vi "HV_Analyse.vi"() -> ()   [LabVIEW 2018]
uses:
  <vilib>/Utility/file.llb/Read Delimited Spreadsheet (string).vi
  <vilib>/Analysis/NI_AALPro.lvlib
panel:
  in  "Main":T1(tab)
  in  "Sow_Median_L1":bool caption="Checkbox"
  out "Progress":dbl(slide) scale=0.0..100.0
  in  "Start":bool
  in  "File path":path
  in  "Threshold [uA]":dbl=0.05
  in  "Window size [min]":dbl=2.0 min=2.0 max=180.0 step=1.0
  in  "Stop":bool
  out "L1-Voltage":cluster{timestamp[], dbl[]}[](graph)
  out "L1-Current [uA]":T2(graph)
  out "L1-Average/WindowSize":T3(graph)
  out "L1-Sparks/min":T4(graph)
  in  "Sow_Median_L2":bool caption="Checkbox"
  out "L2-Sparks/min":T4(graph)
  out "L2-Average/WindowSize":T3(graph)
  out "L2-Current [uA]":T2(graph)
  out "L2-Voltage":cluster{timestamp[], dbl[]}[](graph)
  in  "Sow_Median_L3":bool caption="Checkbox"
  out "L3-Voltage":cluster{timestamp[], dbl[]}[](graph)
  out "L3-Current [uA]":T2(graph)
  out "L3-Average/WindowSize":T3(graph)
  out "L3-Sparks/min":T4(graph)
  in  "Sow_Median_L4":bool caption="Checkbox"
  out "L4-Sparks/min":T4(graph)
  out "L4-Average/WindowSize":T3(graph)
  out "L4-Current [uA]":T2(graph)
  out "L4-Voltage":cluster{timestamp[], dbl[]}[](graph)
  out "Spark-rate statistic_L4":T5(graph) caption="XY Graph - Dark"
  out "Spark-rate statistic_L3":T5(graph) caption="XY Graph - Dark"
  out "Spark-rate statistic_L2":T5(graph) caption="XY Graph - Dark"
  out "Spark-rate statistic_L1":T5(graph) caption="XY Graph - Dark"
  in  "L4_Vertical Slider":cluster{"Slider":dbl, "Slider":dbl}(slide)={"Slider"=0.0, "Slider"=6.702127659574468} scale=-0.25..1.0
  in  "L4_Horizontal Slider":cluster{"Slider":dbl, "Slider":dbl}(slide)={"Slider"=0.0, "Slider"=2.46031746031746} scale=3644665200.0..3644907785.0 scale format="%<%H:%M:%S>T"
  out "L4-Current_Zoomed":cluster{timestamp[], dbl[]}[](graph)
  out "L4-Current_Full":cluster{timestamp[], dbl[]}[](graph)
  in  "L3_Vertical Slider":cluster{"Slider":dbl, "Slider":dbl}(slide)={"Slider"=0.0, "Slider"=6.702127659574468} scale=-1.0..3.0
  in  "L3_Horizontal Slider":cluster{"Slider":dbl, "Slider":dbl}(slide)={"Slider"=0.0, "Slider"=2.46031746031746} scale=3644665200.0..3644907785.0 scale format="%<%H:%M:%S>T"
  out "L3-Current_Zoomed":cluster{timestamp[], dbl[]}[](graph)
  out "L3-Current_Full":cluster{timestamp[], dbl[]}[](graph)
  in  "L2_Vertical Slider":cluster{"Slider":dbl, "Slider":dbl}(slide)={"Slider"=0.0, "Slider"=6.702127659574468} scale=-50.0..100.0
  in  "L2_Horizontal Slider":cluster{"Slider":dbl, "Slider":dbl}(slide)={"Slider"=0.0, "Slider"=2.46031746031746} scale=3644665200.0..3644907785.0 scale format="%<%H:%M:%S>T"
  out "L2-Current_Zoomed":cluster{timestamp[], dbl[]}[](graph)
  out "L2-Current_Full":cluster{timestamp[], dbl[]}[](graph)
  in  "L1_Vertical Slider":cluster{"Slider":dbl, "Slider":dbl}(slide)={"Slider"=0.0, "Slider"=6.702127659574468} scale=-0.2..0.8 scale format="%#_3f"
  in  "L1_Horizontal Slider":cluster{"Slider":dbl, "Slider":dbl}(slide)={"Slider"=0.0, "Slider"=2.46031746031746} scale=3644665200.0..3644907785.0 scale format="%<%H:%M:%S>T"
  out "L1-Current_Zoomed":cluster{timestamp[], dbl[]}[](graph)
  out "L1-Current_Full":cluster{timestamp[], dbl[]}[](graph)
  # "%"
  # "show Median"
  # "show Median"
  # "show Median"
  # "show Median"
  # "Current [uA]"
  # "Current [uA]"
  # "Time"
  # "Time"
  # "Current [uA]"
  # "Current [uA]"
  # "Time"
  # "Time"
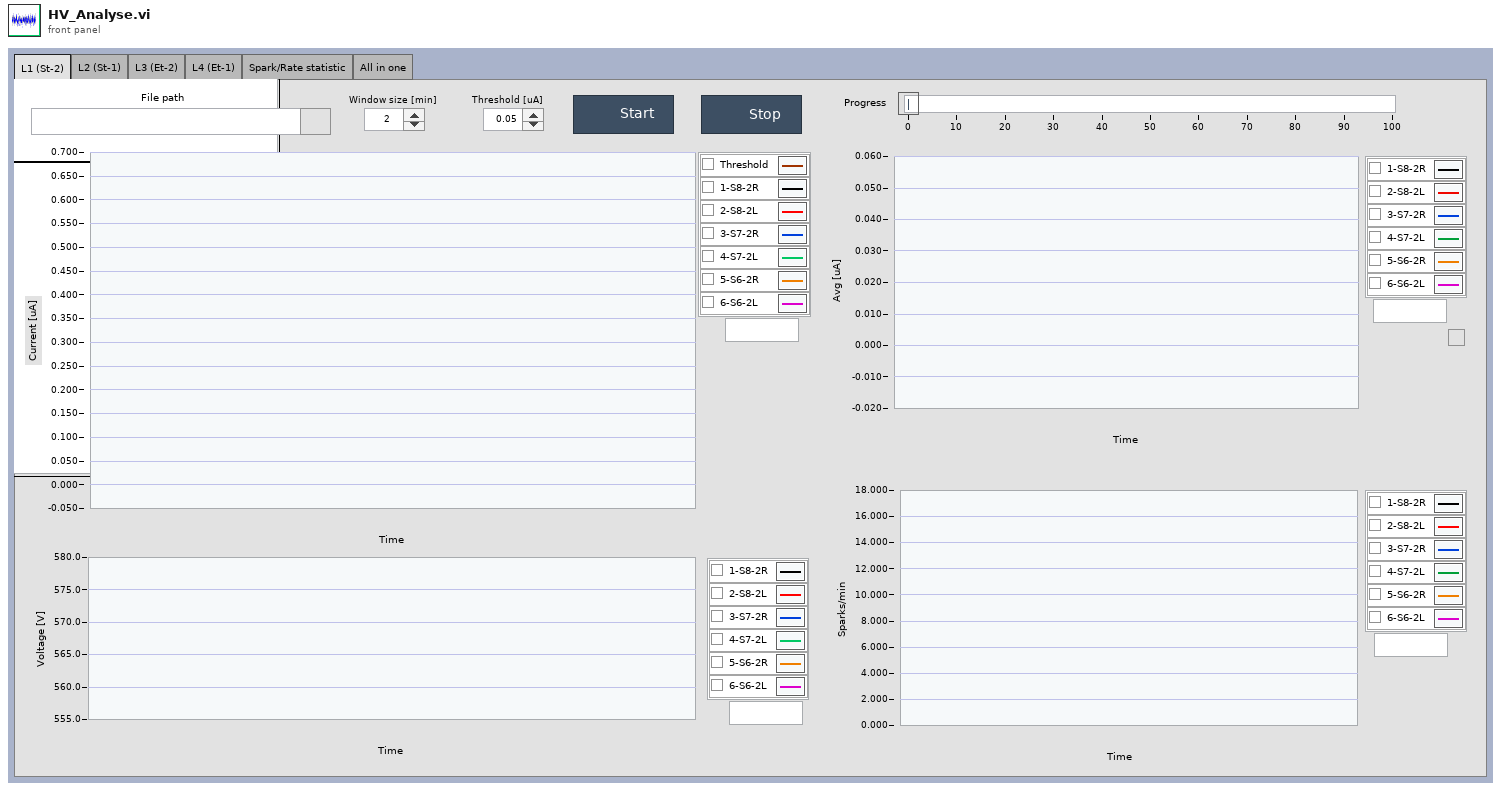
[diagram p1: front panel]
types:
  T1 = enum32{"L1 (St-2)", "L2 (St-1)", "L3 (Et-2)", "L4 (Et-1)", "Spark/Rate statistic", "All in one"}
  T2 = cluster{"Time_Stamp":timestamp[], "Current_Out":dbl[]}[]
  T3 = cluster{"Time_Out":timestamp[], "Window_Avg_OUT":dbl[]}[]
  T4 = cluster{"Time_Out":timestamp[], "Window_Spark_Rate_OUT":dbl[]}[]
  T5 = cluster{"X Values":dbl[], "Histogram: h(x)":i32[]}[]
  T6 = typedef "LVDateTimeRec.ctl" = cluster{"fractional second":dbl, "second":i32, "minute":i32, "hour":i32, "day of month":i32, "month":i32, "year":i32, "day of week":i32, "day of year":i32, "DST":i32}
  T7 = cluster{dbl, i32, i32, i32, "day of month":i32, "month":i32, "year":i32, "day of week":i32, "day of year":i32, "DST":i32}
  T8 = cluster{"XScale.Maximum":dbl, "XScale.Minimum":dbl}
  T9 = cluster{"YScale.Maximum":dbl, "YScale.Minimum":dbl}
  T10 = cluster{"X Values":dbl[], "Histogram: h(x)":i32[]}
  T11 = cluster{"Time_Out":timestamp[], "Window_Avg_OUT":dbl[]}
  T12 = cluster{"Time_Out":timestamp[], "Window_Spark_Rate_OUT":dbl[]}
  T13 = cluster{"Time_Out":timestamp[], "Window_Median_OUT":dbl[]}
  T14 = cluster{"Time_Out":timestamp[], "Window_Median_OUT":dbl[]}[]
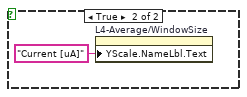
[diagram p3: hidden frame]
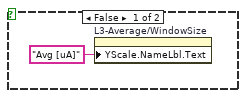
[diagram p4: hidden frame]
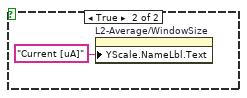
[diagram p5: hidden frame]
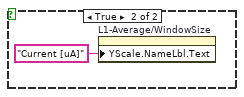
[diagram p6: hidden frame]
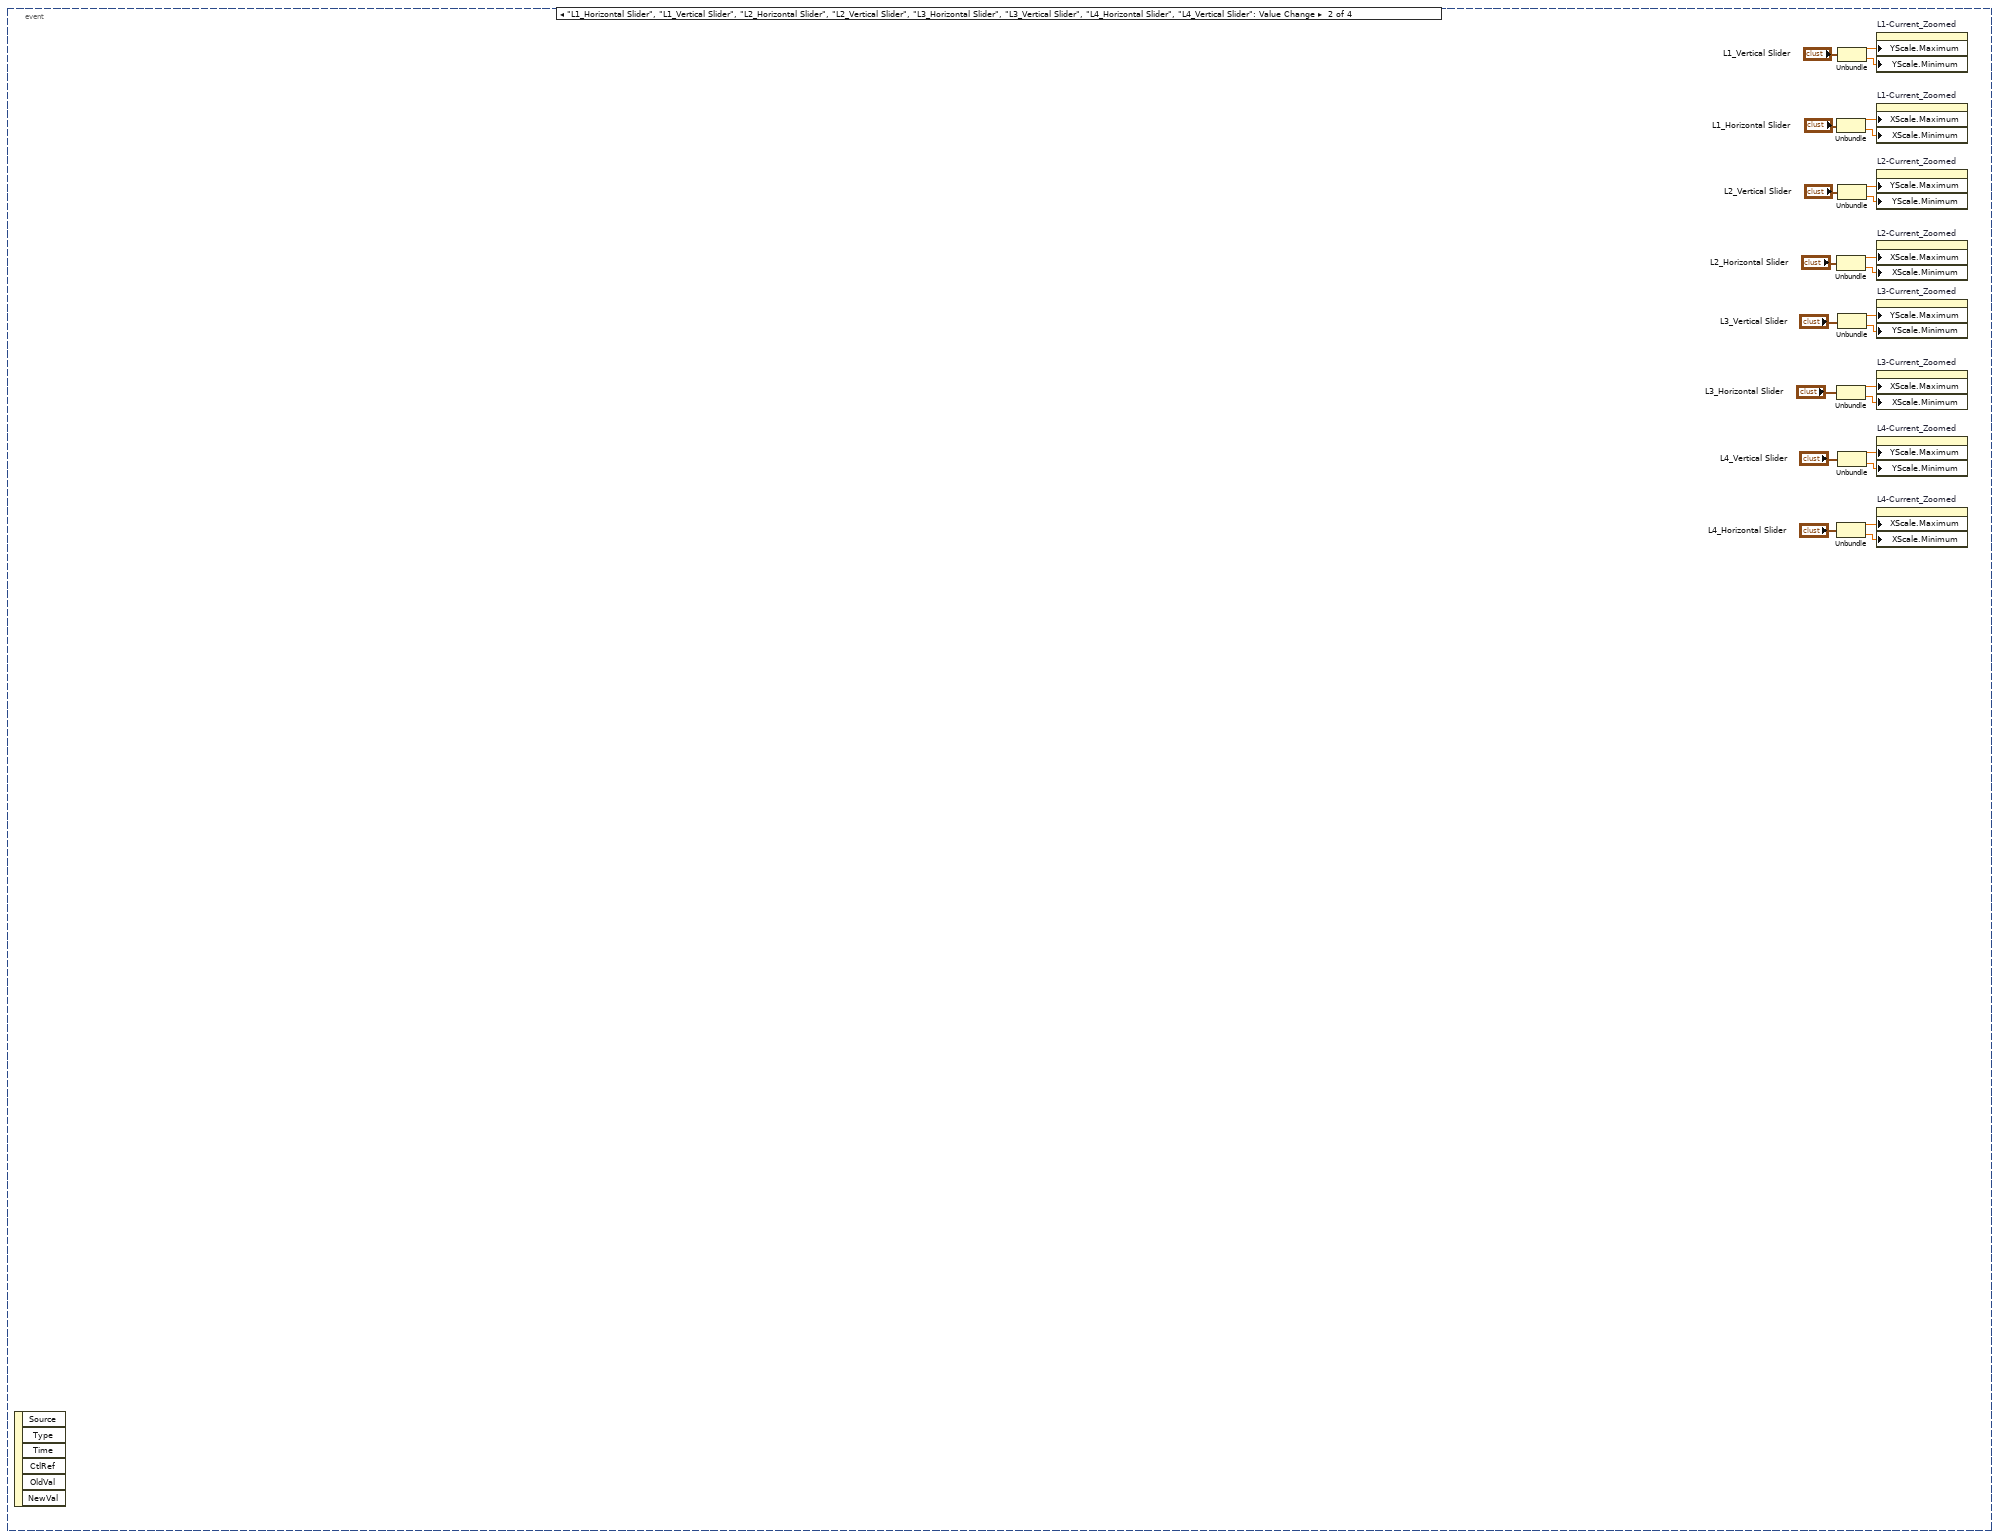
[diagram p7: hidden frame]
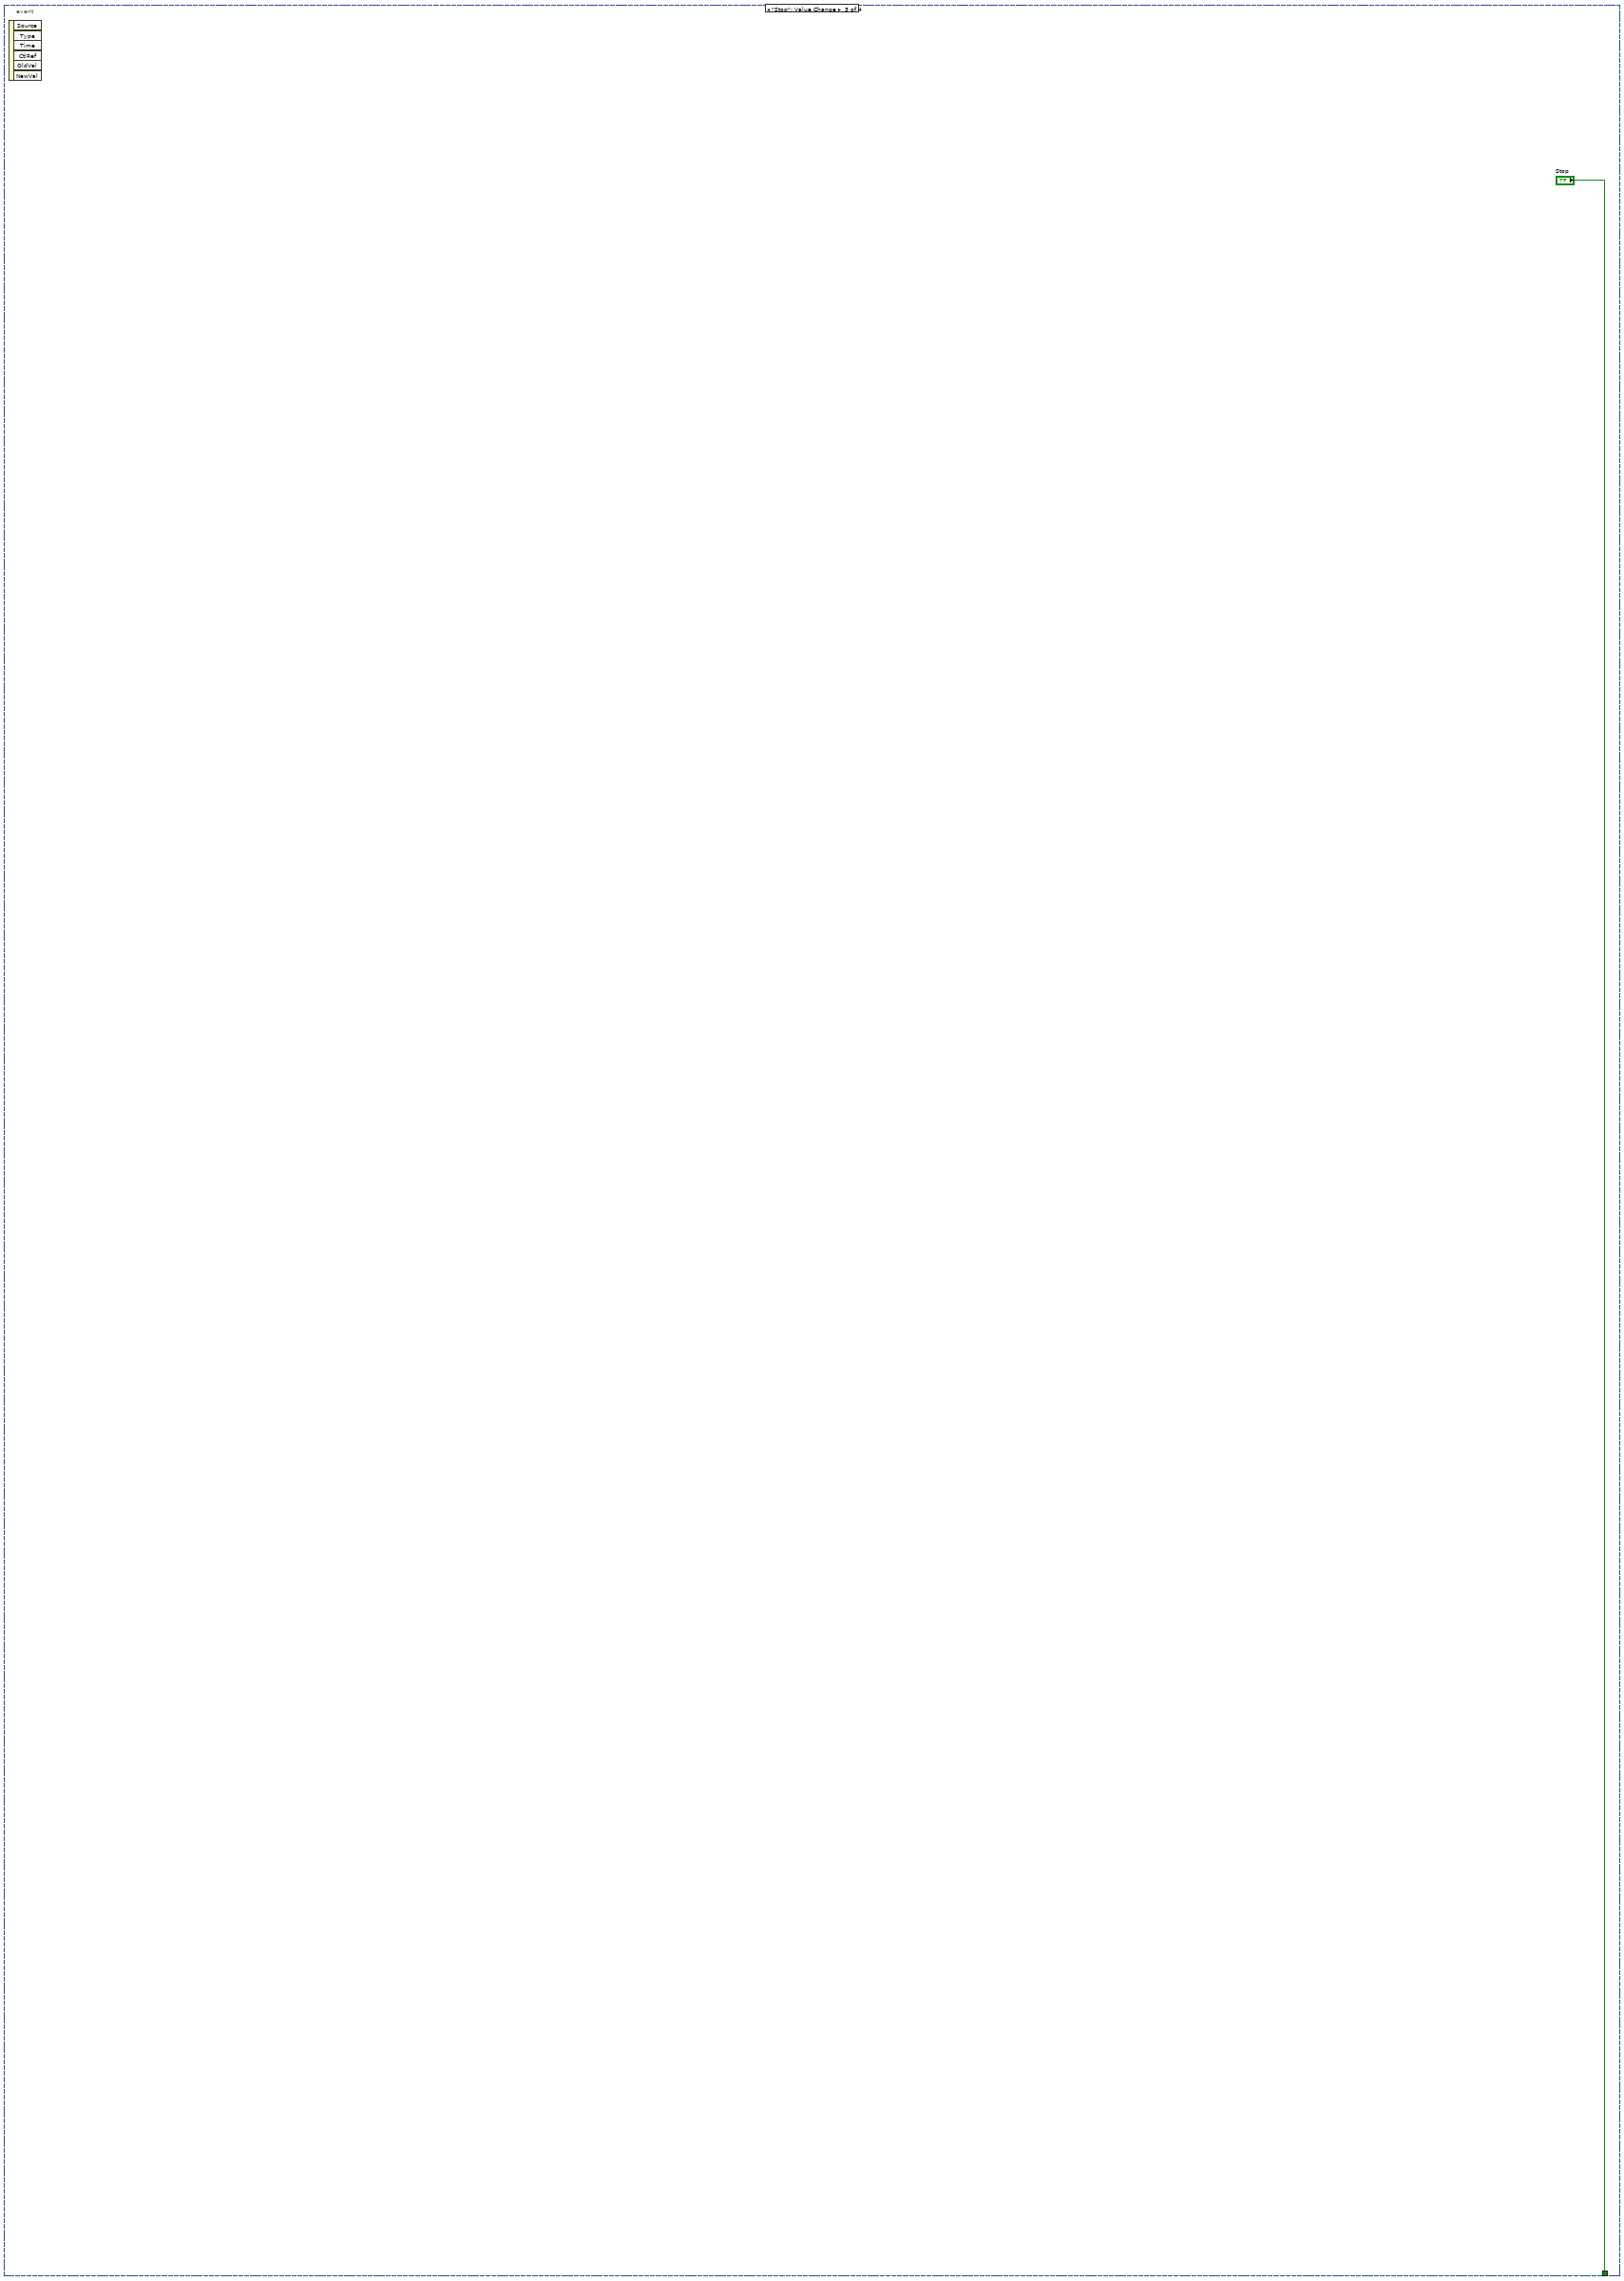
[diagram p8: hidden frame]
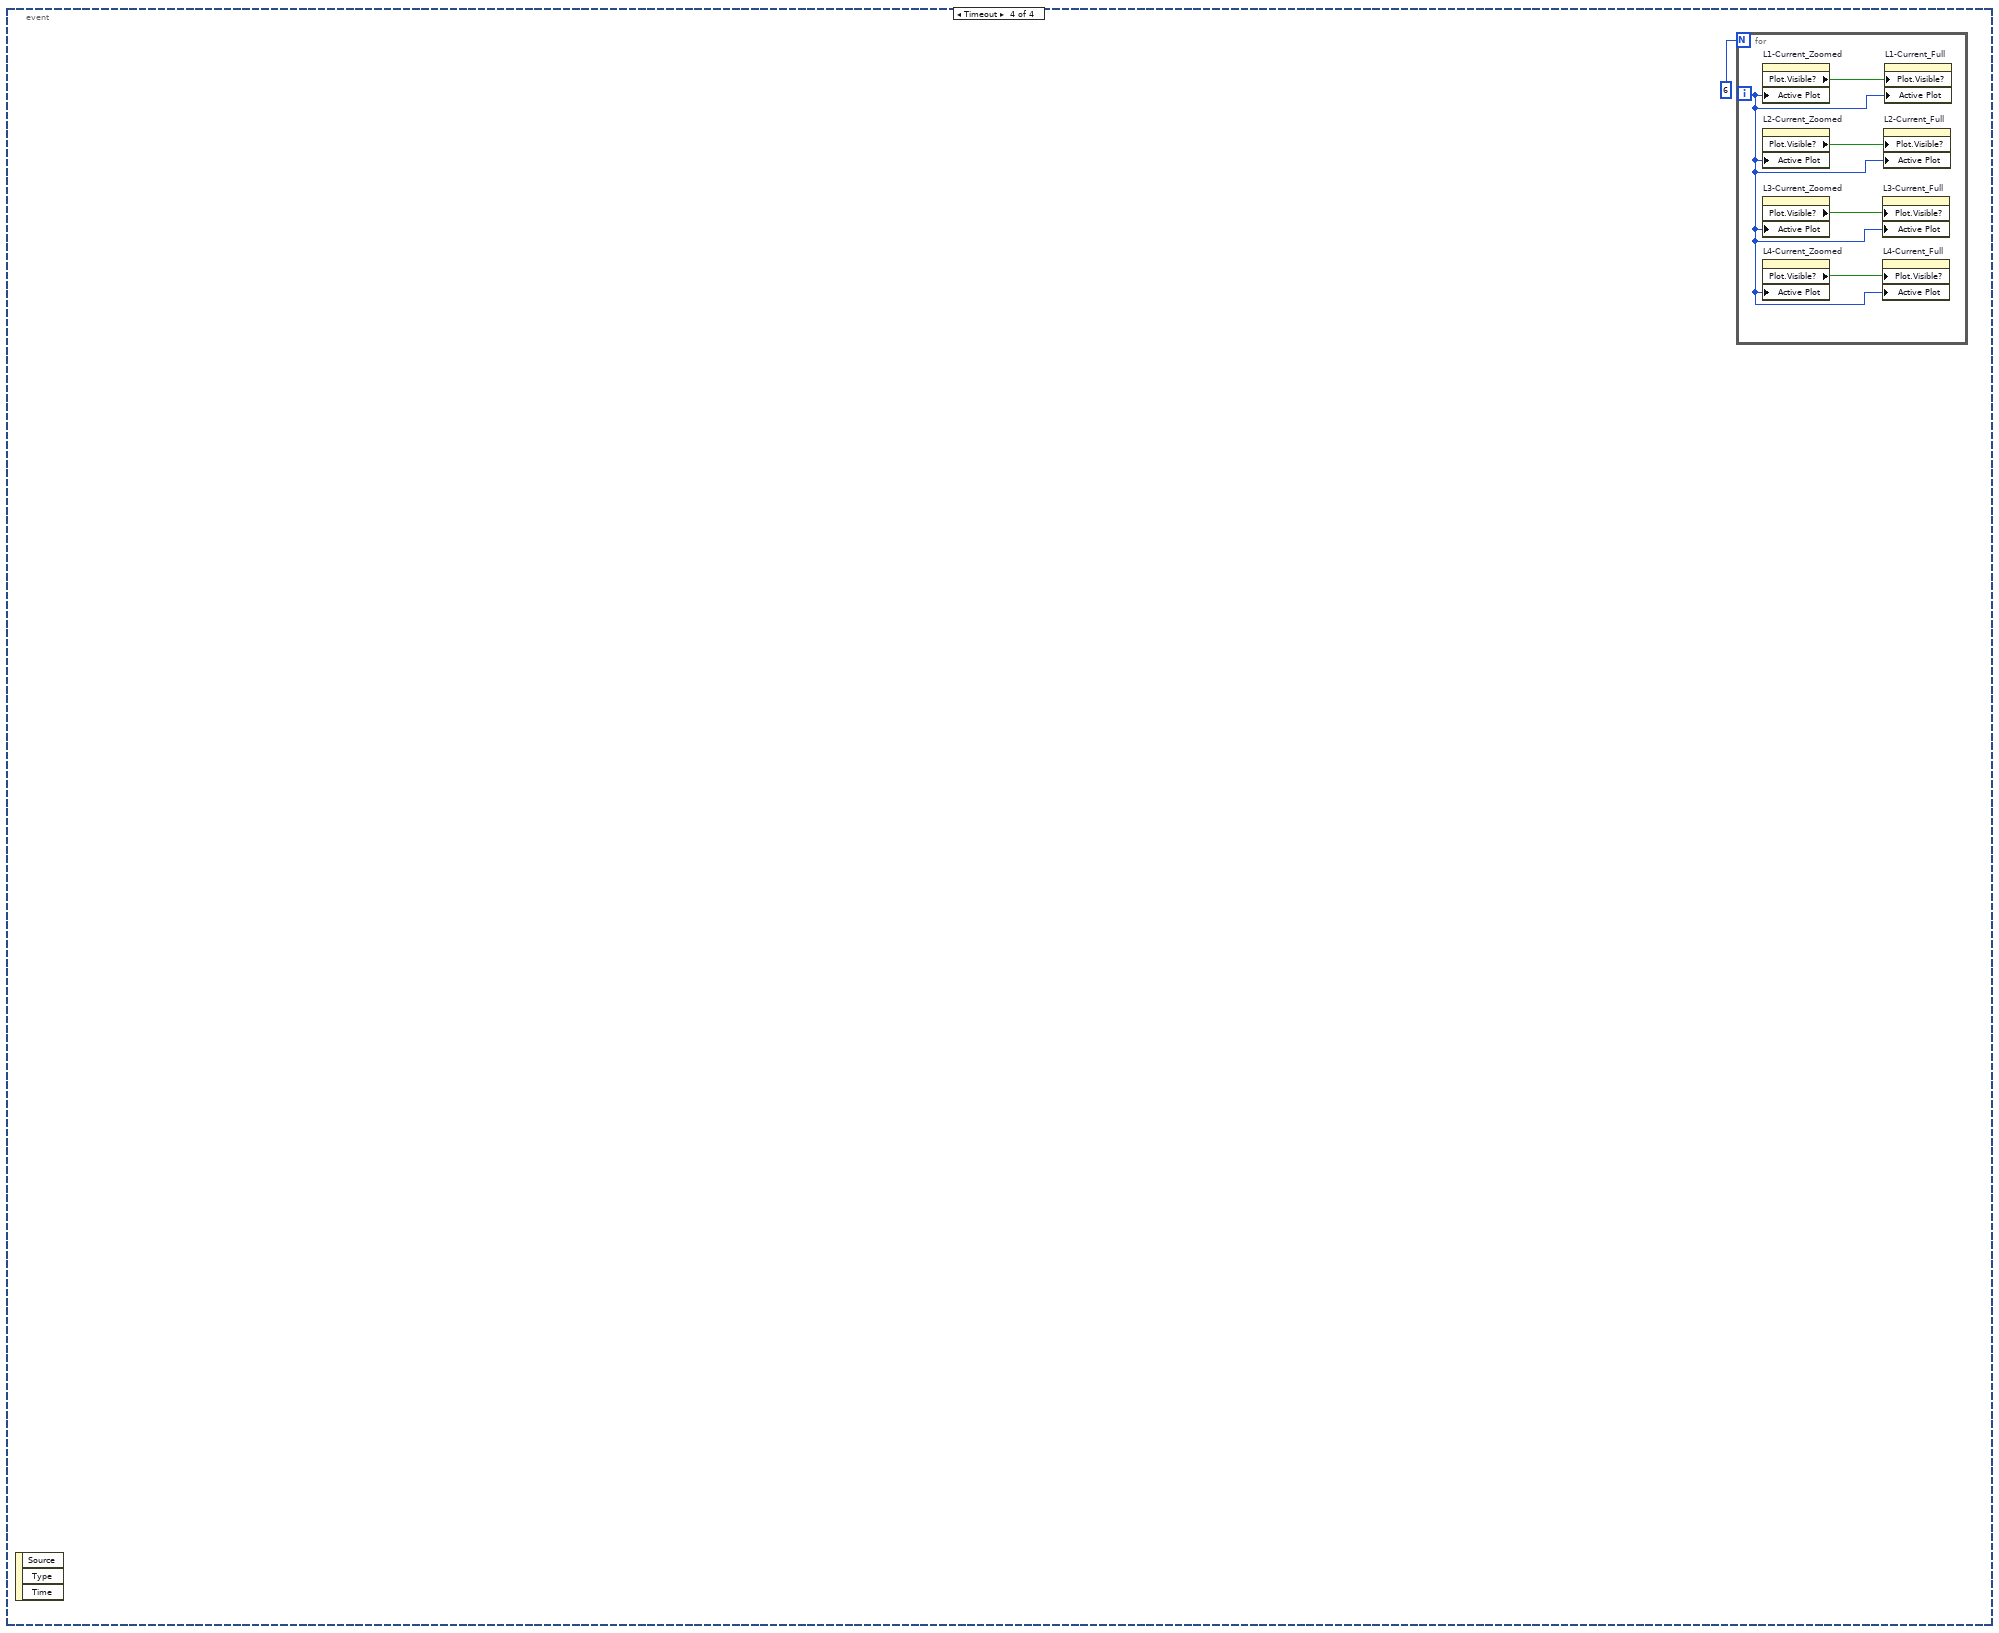
[diagram p9: hidden frame]
diagram:
  n1 = while {
    stop <- w1 stop-if-true
    n2 = event shown="[0] \"Start\", \"Sow_Median_L1\", \"Sow_Median_L2\", \"Sow_Median_L3\", \"Sow_Median_L4\": Value Change" {
      selector: _ -> [_ _ _ _]
      dyn-events: _ -> [_ _ _ _]
      timeout: 400 -> [_ _ _ _]
      tunnel: [_ _ "Stop" _] -> w1
      event "Start", "Sow_Median_L1", "Sow_Median_L2", "Sow_Median_L3", "Sow_Median_L4": Value Change {
        w385 = 31 ("# bins")
        w387 = 0.0 ("min")
        w386 = 6.2 ("max")
        w412 = 31 ("# bins")
        w410 = 0.0 ("min")
        w411 = 6.2 ("max")
        w683 = 0
        # "Amount of windows size"
        # "Full time in minute"
        # "Full time in seconds"
        # "First time stamp"
        # "Last time stamp"
        # "Ch24"
        # "Ch23"
        # "Ch22"
        # "Ch21"
        # "Ch20"
        # "Ch19"
        # "Ch18"
        # "Ch17"
        # "Ch16"
        # "Ch15"
        # "Ch14"
        # "Ch13"
        # "Ch12"
        # "Ch11"
        # "Ch10"
        # "Ch9"
        # "Ch8"
        # "Ch7"
        # "Ch6"
        # "Ch5"
        # "Ch4"
        # "Ch3"
        # "Ch2"
        # "Ch1"
        # "Ch19-Ch24\nCurrent"
        # "Ch13-Ch18\nCurrent"
        # "Ch7-Ch12\nCurrent"
        # "Ch1-Ch6\nCurrent"
        # "Graphs for slider\nmanipulation"
        # "Time Stamp array"
        # "Threshold Graph\nIndicator"
        # "Vlotage Graphs"
        # "L4"
        # "L3"
        # "L2"
        # "L1"
        n3 = event-data() -> ()  [unwired: 1 in, 6 out]
        n4 = call-poly <vilib>:"Read Delimited Spreadsheet.vi"("file path (dialog if empty)"="File path") -> ("all rows"=w112:string[][])  [unwired: 9 in, 5 out]
        n5 = Index Array(array=w112, index (col)=0 ("disabled index (col)")) -> (element=w354:string[])  [unwired: 1 in]
        n6 = Index Array(array=w112, index (col)=1 ("disabled index (col)")) -> (element=w350:string[])  [unwired: 1 in]
        n7 = Index Array(array=w112, index (col)=2 ("disabled index (col)")) -> (element=w345:string[])  [unwired: 1 in]
        n8 = Index Array(array=w112, index (col)=5 ("disabled index (col)")) -> (element=w316:string[])  [unwired: 1 in]
        n9 = Index Array(array=w112, index (col)=6 ("disabled index (col)")) -> (element=w321:string[])  [unwired: 1 in]
        n10 = Index Array(array=w112, index (col)=15 ("disabled index (col)")) -> (element=w275:string[])  [unwired: 1 in]
        n11 = Index Array(array=w112, index (col)=16 ("disabled index (col)")) -> (element=w280:string[])  [unwired: 1 in]
        n12 = Index Array(array=w112, index (col)=25 ("disabled index (col)")) -> (element=w309:string[])  [unwired: 1 in]
        n13 = Index Array(array=w112, index (col)=26 ("disabled index (col)")) -> (element=w304:string[])  [unwired: 1 in]
        n14 = Index Array(array=w112, index (col)=3 ("disabled index (col)")) -> (element=w336:string[])  [unwired: 1 in]
        n15 = Index Array(array=w112, index (col)=4 ("disabled index (col)")) -> (element=w340:string[])  [unwired: 1 in]
        n16 = Index Array(array=w112, index (col)=13 ("disabled index (col)")) -> (element=w331:string[])  [unwired: 1 in]
        n17 = Index Array(array=w112, index (col)=14 ("disabled index (col)")) -> (element=w326:string[])  [unwired: 1 in]
        n18 = Index Array(array=w112, index (col)=17 ("disabled index (col)")) -> (element=w289:string[])  [unwired: 1 in]
        n19 = Index Array(array=w112, index (col)=18 ("disabled index (col)")) -> (element=w285:string[])  [unwired: 1 in]
        n20 = Index Array(array=w112, index (col)=27 ("disabled index (col)")) -> (element=w294:string[])  [unwired: 1 in]
        n21 = Index Array(array=w112, index (col)=28 ("disabled index (col)")) -> (element=w299:string[])  [unwired: 1 in]
        n22 = Index Array(array=w112, index (col)=29 ("disabled index (col)")) -> (element=w270:string[])  [unwired: 1 in]
        n23 = Index Array(array=w112, index (col)=38 ("disabled index (col)")) -> (element=w241:string[])  [unwired: 1 in]
        n24 = Index Array(array=w112, index (col)=39 ("disabled index (col)")) -> (element=w246:string[])  [unwired: 1 in]
        n25 = Index Array(array=w112, index (col)=42 ("disabled index (col)")) -> (element=w235:string[])  [unwired: 1 in]
        n26 = Index Array(array=w112, index (col)=30 ("disabled index (col)")) -> (element=w261:string[])  [unwired: 1 in]
        n27 = Index Array(array=w112, index (col)=37 ("disabled index (col)")) -> (element=w265:string[])  [unwired: 1 in]
        n28 = Index Array(array=w112, index (col)=40 ("disabled index (col)")) -> (element=w256:string[])  [unwired: 1 in]
        n29 = Index Array(array=w112, index (col)=41 ("disabled index (col)")) -> (element=w251:string[])  [unwired: 1 in]
        n30 = Index Array(array=w112, index (col)=7 ("disabled index (col)")) -> (element=w115:string[])  [unwired: 1 in]
        n31 = Index Array(array=w112, index (col)=8 ("disabled index (col)")) -> (element=w120:string[])  [unwired: 1 in]
        n32 = Index Array(array=w112, index (col)=11 ("disabled index (col)")) -> (element=w149:string[])  [unwired: 1 in]
        n33 = Index Array(array=w112, index (col)=12 ("disabled index (col)")) -> (element=w144:string[])  [unwired: 1 in]
        n34 = Index Array(array=w112, index (col)=21 ("disabled index (col)")) -> (element=w190:string[])  [unwired: 1 in]
        n35 = Index Array(array=w112, index (col)=22 ("disabled index (col)")) -> (element=w185:string[])  [unwired: 1 in]
        n36 = Index Array(array=w112, index (col)=31 ("disabled index (col)")) -> (element=w156:string[])  [unwired: 1 in]
        n37 = Index Array(array=w112, index (col)=32 ("disabled index (col)")) -> (element=w161:string[])  [unwired: 1 in]
        n38 = Index Array(array=w112, index (col)=9 ("disabled index (col)")) -> (element=w129:string[])  [unwired: 1 in]
        n39 = Index Array(array=w112, index (col)=10 ("disabled index (col)")) -> (element=w125:string[])  [unwired: 1 in]
        n40 = Index Array(array=w112, index (col)=19 ("disabled index (col)")) -> (element=w134:string[])  [unwired: 1 in]
        n41 = Index Array(array=w112, index (col)=20 ("disabled index (col)")) -> (element=w139:string[])  [unwired: 1 in]
        n42 = Index Array(array=w112, index (col)=23 ("disabled index (col)")) -> (element=w176:string[])  [unwired: 1 in]
        n43 = Index Array(array=w112, index (col)=24 ("disabled index (col)")) -> (element=w180:string[])  [unwired: 1 in]
        n44 = Index Array(array=w112, index (col)=33 ("disabled index (col)")) -> (element=w171:string[])  [unwired: 1 in]
        n45 = Index Array(array=w112, index (col)=34 ("disabled index (col)")) -> (element=w166:string[])  [unwired: 1 in]
        n46 = Index Array(array=w112, index (col)=35 ("disabled index (col)")) -> (element=w195:string[])  [unwired: 1 in]
        n47 = Index Array(array=w112, index (col)=44 ("disabled index (col)")) -> (element=w224:string[])  [unwired: 1 in]
        n48 = Index Array(array=w112, index (col)=45 ("disabled index (col)")) -> (element=w219:string[])  [unwired: 1 in]
        n49 = Index Array(array=w112, index (col)=48 ("disabled index (col)")) -> (element=w230:string[])  [unwired: 1 in]
        n50 = Index Array(array=w112, index (col)=36 ("disabled index (col)")) -> (element=w204:string[])  [unwired: 1 in]
        n51 = Index Array(array=w112, index (col)=43 ("disabled index (col)")) -> (element=w200:string[])  [unwired: 1 in]
        n52 = Index Array(array=w112, index (col)=46 ("disabled index (col)")) -> (element=w209:string[])  [unwired: 1 in]
        n53 = Index Array(array=w112, index (col)=47 ("disabled index (col)")) -> (element=w214:string[])  [unwired: 1 in]
        n54 = Delete From Array(array=w350, length=2, index=0) -> (array with subset deleted=w348:string[])  [unwired: 1 out]
        n55 = Delete From Array(array=w345, length=2, index=0) -> (array with subset deleted=w347:string[])  [unwired: 1 out]
        n56 = Delete From Array(array=w316, length=2, index=0) -> (array with subset deleted=w318:string[])  [unwired: 1 out]
        n57 = Delete From Array(array=w321, length=2, index=0) -> (array with subset deleted=w319:string[])  [unwired: 1 out]
        n58 = Delete From Array(array=w275, length=2, index=0) -> (array with subset deleted=w277:string[])  [unwired: 1 out]
        n59 = Delete From Array(array=w280, length=2, index=0) -> (array with subset deleted=w278:string[])  [unwired: 1 out]
        n60 = Delete From Array(array=w309, length=2, index=0) -> (array with subset deleted=w307:string[])  [unwired: 1 out]
        n61 = Delete From Array(array=w304, length=2, index=0) -> (array with subset deleted=w306:string[])  [unwired: 1 out]
        n62 = Delete From Array(array=w354, length=2, index=0) -> (array with subset deleted=w353:string[])  [unwired: 1 out]
        n63 = Delete From Array(array=w336, length=2, index=0) -> (array with subset deleted=w338:string[])  [unwired: 1 out]
        n64 = Delete From Array(array=w340, length=2, index=0) -> (array with subset deleted=w339:string[])  [unwired: 1 out]
        n65 = Delete From Array(array=w331, length=2, index=0) -> (array with subset deleted=w329:string[])  [unwired: 1 out]
        n66 = Delete From Array(array=w326, length=2, index=0) -> (array with subset deleted=w328:string[])  [unwired: 1 out]
        n67 = Delete From Array(array=w289, length=2, index=0) -> (array with subset deleted=w287:string[])  [unwired: 1 out]
        n68 = Delete From Array(array=w285, length=2, index=0) -> (array with subset deleted=w286:string[])  [unwired: 1 out]
        n69 = Delete From Array(array=w294, length=2, index=0) -> (array with subset deleted=w296:string[])  [unwired: 1 out]
        n70 = Delete From Array(array=w299, length=2, index=0) -> (array with subset deleted=w297:string[])  [unwired: 1 out]
        n71 = Delete From Array(array=w270, length=2, index=0) -> (array with subset deleted=w272:string[])  [unwired: 1 out]
        n72 = Delete From Array(array=w241, length=2, index=0) -> (array with subset deleted=w243:string[])  [unwired: 1 out]
        n73 = Delete From Array(array=w246, length=2, index=0) -> (array with subset deleted=w244:string[])  [unwired: 1 out]
        n74 = Delete From Array(array=w235, length=2, index=0) -> (array with subset deleted=w233:string[])  [unwired: 1 out]
        n75 = Delete From Array(array=w261, length=2, index=0) -> (array with subset deleted=w263:string[])  [unwired: 1 out]
        n76 = Delete From Array(array=w265, length=2, index=0) -> (array with subset deleted=w264:string[])  [unwired: 1 out]
        n77 = Delete From Array(array=w256, length=2, index=0) -> (array with subset deleted=w254:string[])  [unwired: 1 out]
        n78 = Delete From Array(array=w251, length=2, index=0) -> (array with subset deleted=w253:string[])  [unwired: 1 out]
        n79 = Delete From Array(array=w115, length=2, index=0) -> (array with subset deleted=w117:string[])  [unwired: 1 out]
        n80 = Delete From Array(array=w120, length=2, index=0) -> (array with subset deleted=w118:string[])  [unwired: 1 out]
        n81 = Delete From Array(array=w149, length=2, index=0) -> (array with subset deleted=w147:string[])  [unwired: 1 out]
        n82 = Delete From Array(array=w144, length=2, index=0) -> (array with subset deleted=w146:string[])  [unwired: 1 out]
        n83 = Delete From Array(array=w190, length=2, index=0) -> (array with subset deleted=w188:string[])  [unwired: 1 out]
        n84 = Delete From Array(array=w185, length=2, index=0) -> (array with subset deleted=w187:string[])  [unwired: 1 out]
        n85 = Delete From Array(array=w156, length=2, index=0) -> (array with subset deleted=w158:string[])  [unwired: 1 out]
        n86 = Delete From Array(array=w161, length=2, index=0) -> (array with subset deleted=w159:string[])  [unwired: 1 out]
        n87 = Delete From Array(array=w129, length=2, index=0) -> (array with subset deleted=w127:string[])  [unwired: 1 out]
        n88 = Delete From Array(array=w125, length=2, index=0) -> (array with subset deleted=w126:string[])  [unwired: 1 out]
        n89 = Delete From Array(array=w134, length=2, index=0) -> (array with subset deleted=w136:string[])  [unwired: 1 out]
        n90 = Delete From Array(array=w139, length=2, index=0) -> (array with subset deleted=w137:string[])  [unwired: 1 out]
        n91 = Delete From Array(array=w176, length=2, index=0) -> (array with subset deleted=w178:string[])  [unwired: 1 out]
        n92 = Delete From Array(array=w180, length=2, index=0) -> (array with subset deleted=w179:string[])  [unwired: 1 out]
        n93 = Delete From Array(array=w171, length=2, index=0) -> (array with subset deleted=w169:string[])  [unwired: 1 out]
        n94 = Delete From Array(array=w166, length=2, index=0) -> (array with subset deleted=w168:string[])  [unwired: 1 out]
        n95 = Delete From Array(array=w195, length=2, index=0) -> (array with subset deleted=w193:string[])  [unwired: 1 out]
        n96 = Delete From Array(array=w224, length=2, index=0) -> (array with subset deleted=w222:string[])  [unwired: 1 out]
        n97 = Delete From Array(array=w219, length=2, index=0) -> (array with subset deleted=w221:string[])  [unwired: 1 out]
        n98 = Delete From Array(array=w230, length=2, index=0) -> (array with subset deleted=w232:string[])  [unwired: 1 out]
        n99 = Delete From Array(array=w204, length=2, index=0) -> (array with subset deleted=w202:string[])  [unwired: 1 out]
        n100 = Delete From Array(array=w200, length=2, index=0) -> (array with subset deleted=w201:string[])  [unwired: 1 out]
        n101 = Delete From Array(array=w209, length=2, index=0) -> (array with subset deleted=w211:string[])  [unwired: 1 out]
        n102 = Delete From Array(array=w214, length=2, index=0) -> (array with subset deleted=w212:string[])  [unwired: 1 out]
        n103 = for {
          tunnel: w353 -> [w1164] mode=indexing
          tunnel: [w1163] -> w111 mode=indexing
          n104 = Scan From String(format string="%<%d.%m.%Y %H:%M:%S>T", input string=w1164) -> (output 1=w1163:timestamp)  [unwired: 3 in, 3 out]
        }
        n105 = for {
          tunnel: w348 -> [w1158] mode=indexing
          tunnel: [w917] -> w100 mode=indexing
          tunnel: w347 -> [w1157] mode=indexing
          tunnel: [w912] -> w99 mode=indexing
          tunnel: w338 -> [w1147] mode=indexing
          tunnel: w339 -> [w1148] mode=indexing
          tunnel: [w901] -> w98 mode=indexing
          tunnel: [w899] -> w97 mode=indexing
          tunnel: w318 -> [w1127] mode=indexing
          tunnel: [w876] -> w96 mode=indexing
          tunnel: w319 -> [w1128] mode=indexing
          tunnel: [w877] -> w95 mode=indexing
          tunnel: w329 -> [w1138] mode=indexing
          tunnel: w328 -> [w1137] mode=indexing
          tunnel: [w878] -> w88 mode=indexing
          tunnel: [w875] -> w87 mode=indexing
          tunnel: w277 -> [w1087] mode=indexing
          tunnel: [w841] -> w86 mode=indexing
          tunnel: w278 -> [w1088] mode=indexing
          tunnel: [w827] -> w85 mode=indexing
          tunnel: w287 -> [w1098] mode=indexing
          tunnel: w286 -> [w1097] mode=indexing
          tunnel: [w828] -> w84 mode=indexing
          tunnel: [w829] -> w83 mode=indexing
          tunnel: w307 -> [w1118] mode=indexing
          tunnel: [w830] -> w76 mode=indexing
          tunnel: w306 -> [w1117] mode=indexing
          tunnel: [w831] -> w75 mode=indexing
          tunnel: w296 -> [w1107] mode=indexing
          tunnel: w297 -> [w1108] mode=indexing
          tunnel: [w832] -> w74 mode=indexing
          tunnel: [w833] -> w73 mode=indexing
          tunnel: w272 -> [w1082] mode=indexing
          tunnel: [w797] -> w72 mode=indexing
          tunnel: w263 -> [w1072] mode=indexing
          tunnel: w264 -> [w1073] mode=indexing
          tunnel: [w795] -> w71 mode=indexing
          tunnel: [w794] -> w64 mode=indexing
          tunnel: w243 -> [w1052] mode=indexing
          tunnel: [w793] -> w63 mode=indexing
          tunnel: w244 -> [w1053] mode=indexing
          tunnel: [w792] -> w62 mode=indexing
          tunnel: w254 -> [w1063] mode=indexing
          tunnel: w253 -> [w1062] mode=indexing
          tunnel: [w791] -> w61 mode=indexing
          tunnel: [w779] -> w60 mode=indexing
          tunnel: w233 -> [w1043] mode=indexing
          tunnel: [w780] -> w59 mode=indexing
          tunnel: w117 -> [w927] mode=indexing
          tunnel: [w778] -> w31 mode=indexing
          tunnel: w118 -> [w928] mode=indexing
          tunnel: [w777] -> w30 mode=indexing
          tunnel: w127 -> [w938] mode=indexing
          tunnel: w126 -> [w937] mode=indexing
          tunnel: [w776] -> w29 mode=indexing
          tunnel: [w775] -> w28 mode=indexing
          tunnel: w147 -> [w958] mode=indexing
          tunnel: [w774] -> w27 mode=indexing
          tunnel: w146 -> [w957] mode=indexing
          tunnel: [w773] -> w26 mode=indexing
          tunnel: w136 -> [w947] mode=indexing
          tunnel: w137 -> [w948] mode=indexing
          tunnel: [w772] -> w24 mode=indexing
          tunnel: [w771] -> w23 mode=indexing
          tunnel: w188 -> [w998] mode=indexing
          tunnel: [w770] -> w22 mode=indexing
          tunnel: w187 -> [w997] mode=indexing
          tunnel: [w769] -> w21 mode=indexing
          tunnel: w178 -> [w987] mode=indexing
          tunnel: w179 -> [w988] mode=indexing
          tunnel: [w768] -> w20 mode=indexing
          tunnel: [w767] -> w19 mode=indexing
          tunnel: w158 -> [w967] mode=indexing
          tunnel: [w766] -> w18 mode=indexing
          tunnel: w159 -> [w968] mode=indexing
          tunnel: [w765] -> w17 mode=indexing
          tunnel: w169 -> [w978] mode=indexing
          tunnel: w168 -> [w977] mode=indexing
          tunnel: [w764] -> w16 mode=indexing
          tunnel: [w763] -> w15 mode=indexing
          tunnel: w193 -> [w1003] mode=indexing
          tunnel: [w762] -> w14 mode=indexing
          tunnel: w202 -> [w1013] mode=indexing
          tunnel: w201 -> [w1012] mode=indexing
          tunnel: [w761] -> w13 mode=indexing
          tunnel: [w760] -> w12 mode=indexing
          tunnel: w222 -> [w1033] mode=indexing
          tunnel: [w759] -> w11 mode=indexing
          tunnel: w221 -> [w1032] mode=indexing
          tunnel: [w758] -> w10 mode=indexing
          tunnel: w211 -> [w1022] mode=indexing
          tunnel: w212 -> [w1023] mode=indexing
          tunnel: [w757] -> w9 mode=indexing
          tunnel: [w756] -> w8 mode=indexing
          tunnel: w232 -> [w1042] mode=indexing
          tunnel: [w755] -> w7 mode=indexing
          n106 = Search and Replace String(input string=w1158, search string=",", replace string="." ("replace string (\"\")")) -> (result string=w1159:string)  [unwired: 5 in, 3 out]
          n107 = Search and Replace String(input string=w1157, search string=",", replace string="." ("replace string (\"\")")) -> (result string=w1156:string)  [unwired: 5 in, 3 out]
          n108 = Search and Replace String(input string=w1127, search string=",", replace string="." ("replace string (\"\")")) -> (result string=w1126:string)  [unwired: 5 in, 3 out]
          n109 = Search and Replace String(input string=w1128, search string=",", replace string="." ("replace string (\"\")")) -> (result string=w1129:string)  [unwired: 5 in, 3 out]
          n110 = Search and Replace String(input string=w1087, search string=",", replace string="." ("replace string (\"\")")) -> (result string=w1086:string)  [unwired: 5 in, 3 out]
          n111 = Search and Replace String(input string=w1088, search string=",", replace string="." ("replace string (\"\")")) -> (result string=w1089:string)  [unwired: 5 in, 3 out]
          n112 = Search and Replace String(input string=w1118, search string=",", replace string="." ("replace string (\"\")")) -> (result string=w1119:string)  [unwired: 5 in, 3 out]
          n113 = Search and Replace String(input string=w1117, search string=",", replace string="." ("replace string (\"\")")) -> (result string=w1116:string)  [unwired: 5 in, 3 out]
          n114 = Search and Replace String(input string=w1147, search string=",", replace string="." ("replace string (\"\")")) -> (result string=w1146:string)  [unwired: 5 in, 3 out]
          n115 = Search and Replace String(input string=w1148, search string=",", replace string="." ("replace string (\"\")")) -> (result string=w1149:string)  [unwired: 5 in, 3 out]
          n116 = Search and Replace String(input string=w1138, search string=",", replace string="." ("replace string (\"\")")) -> (result string=w1139:string)  [unwired: 5 in, 3 out]
          n117 = Search and Replace String(input string=w1137, search string=",", replace string="." ("replace string (\"\")")) -> (result string=w1136:string)  [unwired: 5 in, 3 out]
          n118 = Search and Replace String(input string=w1098, search string=",", replace string="." ("replace string (\"\")")) -> (result string=w1099:string)  [unwired: 5 in, 3 out]
          n119 = Search and Replace String(input string=w1097, search string=",", replace string="." ("replace string (\"\")")) -> (result string=w1096:string)  [unwired: 5 in, 3 out]
          n120 = Search and Replace String(input string=w1107, search string=",", replace string="." ("replace string (\"\")")) -> (result string=w1106:string)  [unwired: 5 in, 3 out]
          n121 = Search and Replace String(input string=w1108, search string=",", replace string="." ("replace string (\"\")")) -> (result string=w1109:string)  [unwired: 5 in, 3 out]
          n122 = Search and Replace String(input string=w1082, search string=",", replace string="." ("replace string (\"\")")) -> (result string=w1081:string)  [unwired: 5 in, 3 out]
          n123 = Search and Replace String(input string=w1052, search string=",", replace string="." ("replace string (\"\")")) -> (result string=w1051:string)  [unwired: 5 in, 3 out]
          n124 = Search and Replace String(input string=w1053, search string=",", replace string="." ("replace string (\"\")")) -> (result string=w1054:string)  [unwired: 5 in, 3 out]
          n125 = Search and Replace String(input string=w1043, search string=",", replace string="." ("replace string (\"\")")) -> (result string=w1044:string)  [unwired: 5 in, 3 out]
          n126 = Search and Replace String(input string=w1072, search string=",", replace string="." ("replace string (\"\")")) -> (result string=w1071:string)  [unwired: 5 in, 3 out]
          n127 = Search and Replace String(input string=w1073, search string=",", replace string="." ("replace string (\"\")")) -> (result string=w1074:string)  [unwired: 5 in, 3 out]
          n128 = Search and Replace String(input string=w1063, search string=",", replace string="." ("replace string (\"\")")) -> (result string=w1064:string)  [unwired: 5 in, 3 out]
          n129 = Search and Replace String(input string=w1062, search string=",", replace string="." ("replace string (\"\")")) -> (result string=w1061:string)  [unwired: 5 in, 3 out]
          n130 = Search and Replace String(input string=w927, search string=",", replace string="." ("replace string (\"\")")) -> (result string=w926:string)  [unwired: 5 in, 3 out]
          n131 = Search and Replace String(input string=w928, search string=",", replace string="." ("replace string (\"\")")) -> (result string=w929:string)  [unwired: 5 in, 3 out]
          n132 = Search and Replace String(input string=w958, search string=",", replace string="." ("replace string (\"\")")) -> (result string=w959:string)  [unwired: 5 in, 3 out]
          n133 = Search and Replace String(input string=w957, search string=",", replace string="." ("replace string (\"\")")) -> (result string=w956:string)  [unwired: 5 in, 3 out]
          n134 = Search and Replace String(input string=w998, search string=",", replace string="." ("replace string (\"\")")) -> (result string=w999:string)  [unwired: 5 in, 3 out]
          n135 = Search and Replace String(input string=w997, search string=",", replace string="." ("replace string (\"\")")) -> (result string=w996:string)  [unwired: 5 in, 3 out]
          n136 = Search and Replace String(input string=w967, search string=",", replace string="." ("replace string (\"\")")) -> (result string=w966:string)  [unwired: 5 in, 3 out]
          n137 = Search and Replace String(input string=w968, search string=",", replace string="." ("replace string (\"\")")) -> (result string=w969:string)  [unwired: 5 in, 3 out]
          n138 = Search and Replace String(input string=w938, search string=",", replace string="." ("replace string (\"\")")) -> (result string=w939:string)  [unwired: 5 in, 3 out]
          n139 = Search and Replace String(input string=w937, search string=",", replace string="." ("replace string (\"\")")) -> (result string=w936:string)  [unwired: 5 in, 3 out]
          n140 = Search and Replace String(input string=w947, search string=",", replace string="." ("replace string (\"\")")) -> (result string=w946:string)  [unwired: 5 in, 3 out]
          n141 = Search and Replace String(input string=w948, search string=",", replace string="." ("replace string (\"\")")) -> (result string=w949:string)  [unwired: 5 in, 3 out]
          n142 = Search and Replace String(input string=w987, search string=",", replace string="." ("replace string (\"\")")) -> (result string=w986:string)  [unwired: 5 in, 3 out]
          n143 = Search and Replace String(input string=w988, search string=",", replace string="." ("replace string (\"\")")) -> (result string=w989:string)  [unwired: 5 in, 3 out]
          n144 = Search and Replace String(input string=w978, search string=",", replace string="." ("replace string (\"\")")) -> (result string=w979:string)  [unwired: 5 in, 3 out]
          n145 = Search and Replace String(input string=w977, search string=",", replace string="." ("replace string (\"\")")) -> (result string=w976:string)  [unwired: 5 in, 3 out]
          n146 = Search and Replace String(input string=w1003, search string=",", replace string="." ("replace string (\"\")")) -> (result string=w1004:string)  [unwired: 5 in, 3 out]
          n147 = Search and Replace String(input string=w1033, search string=",", replace string="." ("replace string (\"\")")) -> (result string=w1034:string)  [unwired: 5 in, 3 out]
          n148 = Search and Replace String(input string=w1032, search string=",", replace string="." ("replace string (\"\")")) -> (result string=w1031:string)  [unwired: 5 in, 3 out]
          n149 = Search and Replace String(input string=w1042, search string=",", replace string="." ("replace string (\"\")")) -> (result string=w1041:string)  [unwired: 5 in, 3 out]
          n150 = Search and Replace String(input string=w1013, search string=",", replace string="." ("replace string (\"\")")) -> (result string=w1014:string)  [unwired: 5 in, 3 out]
          n151 = Search and Replace String(input string=w1012, search string=",", replace string="." ("replace string (\"\")")) -> (result string=w1011:string)  [unwired: 5 in, 3 out]
          n152 = Search and Replace String(input string=w1022, search string=",", replace string="." ("replace string (\"\")")) -> (result string=w1021:string)  [unwired: 5 in, 3 out]
          n153 = Search and Replace String(input string=w1023, search string=",", replace string="." ("replace string (\"\")")) -> (result string=w1024:string)  [unwired: 5 in, 3 out]
          n154 = Fract/Exp String To Number(use system decimal point (T)=FALSE, string=w1159) -> (number=w918:dbl)  [unwired: 2 in, 1 out]
          n155 = Fract/Exp String To Number(use system decimal point (T)=FALSE, string=w1156) -> (number=w911:dbl)  [unwired: 2 in, 1 out]
          n156 = Fract/Exp String To Number(use system decimal point (T)=FALSE, string=w1126) -> (number=w882:dbl)  [unwired: 2 in, 1 out]
          n157 = Fract/Exp String To Number(use system decimal point (T)=FALSE, string=w1129) -> (number=w881:dbl)  [unwired: 2 in, 1 out]
          n158 = Fract/Exp String To Number(use system decimal point (T)=FALSE, string=w1086) -> (number=w842:dbl)  [unwired: 2 in, 1 out]
          n159 = Fract/Exp String To Number(use system decimal point (T)=FALSE, string=w1089) -> (number=w840:dbl)  [unwired: 2 in, 1 out]
          n160 = Fract/Exp String To Number(use system decimal point (T)=FALSE, string=w1119) -> (number=w837:dbl)  [unwired: 2 in, 1 out]
          n161 = Fract/Exp String To Number(use system decimal point (T)=FALSE, string=w1116) -> (number=w836:dbl)  [unwired: 2 in, 1 out]
          n162 = Fract/Exp String To Number(use system decimal point (T)=FALSE, string=w1146) -> (number=w902:dbl)  [unwired: 2 in, 1 out]
          n163 = Fract/Exp String To Number(use system decimal point (T)=FALSE, string=w1149) -> (number=w900:dbl)  [unwired: 2 in, 1 out]
          n164 = Fract/Exp String To Number(use system decimal point (T)=FALSE, string=w1139) -> (number=w880:dbl)  [unwired: 2 in, 1 out]
          n165 = Fract/Exp String To Number(use system decimal point (T)=FALSE, string=w1136) -> (number=w879:dbl)  [unwired: 2 in, 1 out]
          n166 = Fract/Exp String To Number(use system decimal point (T)=FALSE, string=w1099) -> (number=w839:dbl)  [unwired: 2 in, 1 out]
          n167 = Fract/Exp String To Number(use system decimal point (T)=FALSE, string=w1096) -> (number=w838:dbl)  [unwired: 2 in, 1 out]
          n168 = Fract/Exp String To Number(use system decimal point (T)=FALSE, string=w1106) -> (number=w835:dbl)  [unwired: 2 in, 1 out]
          n169 = Fract/Exp String To Number(use system decimal point (T)=FALSE, string=w1109) -> (number=w834:dbl)  [unwired: 2 in, 1 out]
          n170 = Fract/Exp String To Number(use system decimal point (T)=FALSE, string=w1081) -> (number=w802:dbl)  [unwired: 2 in, 1 out]
          n171 = Fract/Exp String To Number(use system decimal point (T)=FALSE, string=w1051) -> (number=w800:dbl)  [unwired: 2 in, 1 out]
          n172 = Fract/Exp String To Number(use system decimal point (T)=FALSE, string=w1054) -> (number=w799:dbl)  [unwired: 2 in, 1 out]
          n173 = Fract/Exp String To Number(use system decimal point (T)=FALSE, string=w1044) -> (number=w781:dbl)  [unwired: 2 in, 1 out]
          n174 = Fract/Exp String To Number(use system decimal point (T)=FALSE, string=w1071) -> (number=w796:dbl)  [unwired: 2 in, 1 out]
          n175 = Fract/Exp String To Number(use system decimal point (T)=FALSE, string=w1074) -> (number=w801:dbl)  [unwired: 2 in, 1 out]
          n176 = Fract/Exp String To Number(use system decimal point (T)=FALSE, string=w1064) -> (number=w798:dbl)  [unwired: 2 in, 1 out]
          n177 = Fract/Exp String To Number(use system decimal point (T)=FALSE, string=w1061) -> (number=w782:dbl)  [unwired: 2 in, 1 out]
          n178 = Fract/Exp String To Number(use system decimal point (T)=FALSE, string=w926) -> (number=w778:dbl)  [unwired: 2 in, 1 out]
          n179 = Fract/Exp String To Number(use system decimal point (T)=FALSE, string=w929) -> (number=w777:dbl)  [unwired: 2 in, 1 out]
          n180 = Fract/Exp String To Number(use system decimal point (T)=FALSE, string=w959) -> (number=w774:dbl)  [unwired: 2 in, 1 out]
          n181 = Fract/Exp String To Number(use system decimal point (T)=FALSE, string=w956) -> (number=w773:dbl)  [unwired: 2 in, 1 out]
          n182 = Fract/Exp String To Number(use system decimal point (T)=FALSE, string=w999) -> (number=w770:dbl)  [unwired: 2 in, 1 out]
          n183 = Fract/Exp String To Number(use system decimal point (T)=FALSE, string=w996) -> (number=w769:dbl)  [unwired: 2 in, 1 out]
          n184 = Fract/Exp String To Number(use system decimal point (T)=FALSE, string=w966) -> (number=w766:dbl)  [unwired: 2 in, 1 out]
          n185 = Fract/Exp String To Number(use system decimal point (T)=FALSE, string=w969) -> (number=w765:dbl)  [unwired: 2 in, 1 out]
          n186 = Fract/Exp String To Number(use system decimal point (T)=FALSE, string=w939) -> (number=w776:dbl)  [unwired: 2 in, 1 out]
          n187 = Fract/Exp String To Number(use system decimal point (T)=FALSE, string=w936) -> (number=w775:dbl)  [unwired: 2 in, 1 out]
          n188 = Fract/Exp String To Number(use system decimal point (T)=FALSE, string=w946) -> (number=w772:dbl)  [unwired: 2 in, 1 out]
          n189 = Fract/Exp String To Number(use system decimal point (T)=FALSE, string=w949) -> (number=w771:dbl)  [unwired: 2 in, 1 out]
          n190 = Fract/Exp String To Number(use system decimal point (T)=FALSE, string=w986) -> (number=w768:dbl)  [unwired: 2 in, 1 out]
          n191 = Fract/Exp String To Number(use system decimal point (T)=FALSE, string=w989) -> (number=w767:dbl)  [unwired: 2 in, 1 out]
          n192 = Fract/Exp String To Number(use system decimal point (T)=FALSE, string=w979) -> (number=w764:dbl)  [unwired: 2 in, 1 out]
          n193 = Fract/Exp String To Number(use system decimal point (T)=FALSE, string=w976) -> (number=w763:dbl)  [unwired: 2 in, 1 out]
          n194 = Fract/Exp String To Number(use system decimal point (T)=FALSE, string=w1004) -> (number=w762:dbl)  [unwired: 2 in, 1 out]
          n195 = Fract/Exp String To Number(use system decimal point (T)=FALSE, string=w1034) -> (number=w759:dbl)  [unwired: 2 in, 1 out]
          n196 = Fract/Exp String To Number(use system decimal point (T)=FALSE, string=w1031) -> (number=w758:dbl)  [unwired: 2 in, 1 out]
          n197 = Fract/Exp String To Number(use system decimal point (T)=FALSE, string=w1041) -> (number=w755:dbl)  [unwired: 2 in, 1 out]
          n198 = Fract/Exp String To Number(use system decimal point (T)=FALSE, string=w1014) -> (number=w761:dbl)  [unwired: 2 in, 1 out]
          n199 = Fract/Exp String To Number(use system decimal point (T)=FALSE, string=w1011) -> (number=w760:dbl)  [unwired: 2 in, 1 out]
          n200 = Fract/Exp String To Number(use system decimal point (T)=FALSE, string=w1021) -> (number=w757:dbl)  [unwired: 2 in, 1 out]
          n201 = Fract/Exp String To Number(use system decimal point (T)=FALSE, string=w1024) -> (number=w756:dbl)  [unwired: 2 in, 1 out]
          n202 = Absolute Value(x=w756) -> (abs(x)=w786:dbl)
          n203 = Absolute Value(x=w755) -> (abs(x)=w787:dbl)
          n204 = Absolute Value(x=w762) -> (abs(x)=w822:dbl)
          n205 = Absolute Value(x=w761) -> (abs(x)=w823:dbl)
          n206 = Absolute Value(x=w760) -> (abs(x)=w807:dbl)
          n207 = Absolute Value(x=w759) -> (abs(x)=w808:dbl)
          n208 = Absolute Value(x=w758) -> (abs(x)=w816:dbl)
          n209 = Absolute Value(x=w757) -> (abs(x)=w815:dbl)
          n210 = Absolute Value(x=w770) -> (abs(x)=w846:dbl)
          n211 = Absolute Value(x=w769) -> (abs(x)=w847:dbl)
          n212 = Absolute Value(x=w768) -> (abs(x)=w855:dbl)
          n213 = Absolute Value(x=w767) -> (abs(x)=w854:dbl)
          n214 = Absolute Value(x=w766) -> (abs(x)=w871:dbl)
          n215 = Absolute Value(x=w765) -> (abs(x)=w870:dbl)
          n216 = Absolute Value(x=w764) -> (abs(x)=w862:dbl)
          n217 = Absolute Value(x=w763) -> (abs(x)=w863:dbl)
          n218 = Absolute Value(x=w778) -> (abs(x)=w919:dbl)
          n219 = Absolute Value(x=w777) -> (abs(x)=w916:dbl)
          n220 = Absolute Value(x=w776) -> (abs(x)=w906:dbl)
          n221 = Absolute Value(x=w775) -> (abs(x)=w907:dbl)
          n222 = Absolute Value(x=w774) -> (abs(x)=w886:dbl)
          n223 = Absolute Value(x=w773) -> (abs(x)=w887:dbl)
          n224 = Absolute Value(x=w772) -> (abs(x)=w895:dbl)
          n225 = Absolute Value(x=w771) -> (abs(x)=w894:dbl)
          n226 = Less?(x=w786, y=5.0) -> (x < y?=w784:bool)
          n227 = Less?(x=w787, y=5.0) -> (x < y?=w789:bool)
          n228 = Less?(x=w822, y=5.0) -> (x < y?=w820:bool)
          n229 = Less?(x=w823, y=5.0) -> (x < y?=w825:bool)
          n230 = Less?(x=w807, y=5.0) -> (x < y?=w805:bool)
          n231 = Less?(x=w808, y=5.0) -> (x < y?=w810:bool)
          n232 = Less?(x=w816, y=5.0) -> (x < y?=w818:bool)
          n233 = Less?(x=w815, y=5.0) -> (x < y?=w813:bool)
          n234 = Less?(x=w846, y=5.0) -> (x < y?=w844:bool)
          n235 = Less?(x=w847, y=5.0) -> (x < y?=w849:bool)
          n236 = Less?(x=w855, y=5.0) -> (x < y?=w857:bool)
          n237 = Less?(x=w854, y=5.0) -> (x < y?=w852:bool)
          n238 = Less?(x=w871, y=5.0) -> (x < y?=w873:bool)
          n239 = Less?(x=w870, y=5.0) -> (x < y?=w868:bool)
          n240 = Less?(x=w862, y=5.0) -> (x < y?=w860:bool)
          n241 = Less?(x=w863, y=5.0) -> (x < y?=w865:bool)
          n242 = Less?(x=w919, y=5.0) -> (x < y?=w921:bool)
          n243 = Less?(x=w916, y=5.0) -> (x < y?=w914:bool)
          n244 = Less?(x=w906, y=5.0) -> (x < y?=w904:bool)
          n245 = Less?(x=w907, y=5.0) -> (x < y?=w909:bool)
          n246 = Less?(x=w886, y=5.0) -> (x < y?=w884:bool)
          n247 = Less?(x=w887, y=5.0) -> (x < y?=w889:bool)
          n248 = Less?(x=w895, y=5.0) -> (x < y?=w897:bool)
          n249 = Less?(x=w894, y=5.0) -> (x < y?=w892:bool)
          n250 = Select(t=0.0, s=w784, f=w782) -> (s? t:f=w779:dbl)
          n251 = Select(t=0.0, s=w789, f=w781) -> (s? t:f=w780:dbl)
          n252 = Select(t=0.0, s=w820, f=w802) -> (s? t:f=w797:dbl)
          n253 = Select(t=0.0, s=w825, f=w796) -> (s? t:f=w795:dbl)
          n254 = Select(t=0.0, s=w805, f=w801) -> (s? t:f=w794:dbl)
          n255 = Select(t=0.0, s=w810, f=w800) -> (s? t:f=w793:dbl)
          n256 = Select(t=0.0, s=w818, f=w799) -> (s? t:f=w792:dbl)
          n257 = Select(t=0.0, s=w813, f=w798) -> (s? t:f=w791:dbl)
          n258 = Select(t=0.0, s=w844, f=w842) -> (s? t:f=w841:dbl)
          n259 = Select(t=0.0, s=w849, f=w840) -> (s? t:f=w827:dbl)
          n260 = Select(t=0.0, s=w857, f=w839) -> (s? t:f=w828:dbl)
          n261 = Select(t=0.0, s=w852, f=w838) -> (s? t:f=w829:dbl)
          n262 = Select(t=0.0, s=w873, f=w837) -> (s? t:f=w830:dbl)
          n263 = Select(t=0.0, s=w868, f=w836) -> (s? t:f=w831:dbl)
          n264 = Select(t=0.0, s=w860, f=w835) -> (s? t:f=w832:dbl)
          n265 = Select(t=0.0, s=w865, f=w834) -> (s? t:f=w833:dbl)
          n266 = Select(t=0.0, s=w921, f=w918) -> (s? t:f=w917:dbl)
          n267 = Select(t=0.0, s=w914, f=w911) -> (s? t:f=w912:dbl)
          n268 = Select(t=0.0, s=w904, f=w902) -> (s? t:f=w901:dbl)
          n269 = Select(t=0.0, s=w909, f=w900) -> (s? t:f=w899:dbl)
          n270 = Select(t=0.0, s=w884, f=w882) -> (s? t:f=w876:dbl)
          n271 = Select(t=0.0, s=w889, f=w881) -> (s? t:f=w877:dbl)
          n272 = Select(t=0.0, s=w897, f=w880) -> (s? t:f=w878:dbl)
          n273 = Select(t=0.0, s=w892, f=w879) -> (s? t:f=w875:dbl)
        }
        n274 = case shown="True" TRUE {
          tunnel: w111 -> [w726 w727]
          tunnel: [w726 w728] -> w25
          frame False {
          }
          frame True {
            n275 = for {
              tunnel: [w741] -> w728 mode=indexing
              tunnel: w727 -> [w737]
              tunnel: w727 -> [w729] mode=indexing
              n276 = Index Array(array=w737, index=0) -> (element=w736:timestamp)
              n277 = Seconds To Date/Time(time stamp (now)=w729) -> (date time rec=w751:T6)  [unwired: 1 in]
              n278 = Seconds To Date/Time(time stamp (now)=w736) -> (date time rec=w742:T6)  [unwired: 1 in]
              n279 = Unbundle By Name(w751) -> ("fractional second"=w750:dbl, "second"=w752:i32, "minute"=w753:i32, "hour"=w754:i32, "day of month"=w735:i32, "month"=w734:i32, "year"=w733:i32, "day of week"=w732:i32, "day of year"=w731:i32, "DST"=w730:i32)
              n280 = Unbundle By Name(w742) -> ("fractional second"=w743:dbl, "second"=w744:i32, "minute"=w745:i32, "hour"=w746:i32)  [unwired: 6 out]
              n281 = Subtract(x=w750, y=w743) -> (x-y=w747:dbl)
              n282 = Subtract(x=w752, y=w744) -> (x-y=w748:i32)
              n283 = Subtract(x=w753, y=w745) -> (x-y=w749:i32)
              n284 = Subtract(x=w754, y=w746) -> (x-y=w739:i32)
              n285 = Bundle(w747, w748, w749, w739, "day of month"=w735, "month"=w734, "year"=w733, "day of week"=w732, "day of year"=w731, "DST"=w730) -> (w738:T7)  [unwired: 1 in]
              n286 = Date/Time To Seconds(2:w738) -> (0:w741:timestamp)  [unwired: 1 in]
            }
          }
        }
        n287 = Bundle(w25, w100) -> (w108:cluster{timestamp[], dbl[]})  [unwired: 1 in]
        n288 = Bundle(w25, w99) -> (w107:cluster{timestamp[], dbl[]})  [unwired: 1 in]
        n289 = Bundle(w25, w98) -> (w106:cluster{timestamp[], dbl[]})  [unwired: 1 in]
        n290 = Bundle(w25, w97) -> (w105:cluster{timestamp[], dbl[]})  [unwired: 1 in]
        n291 = Bundle(w25, w96) -> (w104:cluster{timestamp[], dbl[]})  [unwired: 1 in]
        n292 = Bundle(w25, w95) -> (w103:cluster{timestamp[], dbl[]})  [unwired: 1 in]
        n293 = Bundle(w25, w88) -> (w89:cluster{timestamp[], dbl[]})  [unwired: 1 in]
        n294 = Bundle(w25, w87) -> (w90:cluster{timestamp[], dbl[]})  [unwired: 1 in]
        n295 = Bundle(w25, w86) -> (w91:cluster{timestamp[], dbl[]})  [unwired: 1 in]
        n296 = Bundle(w25, w85) -> (w92:cluster{timestamp[], dbl[]})  [unwired: 1 in]
        n297 = Bundle(w25, w84) -> (w93:cluster{timestamp[], dbl[]})  [unwired: 1 in]
        n298 = Bundle(w25, w83) -> (w94:cluster{timestamp[], dbl[]})  [unwired: 1 in]
        n299 = Bundle(w25, w76) -> (w82:cluster{timestamp[], dbl[]})  [unwired: 1 in]
        n300 = Bundle(w25, w75) -> (w81:cluster{timestamp[], dbl[]})  [unwired: 1 in]
        n301 = Bundle(w25, w74) -> (w80:cluster{timestamp[], dbl[]})  [unwired: 1 in]
        n302 = Bundle(w25, w73) -> (w79:cluster{timestamp[], dbl[]})  [unwired: 1 in]
        n303 = Bundle(w25, w72) -> (w78:cluster{timestamp[], dbl[]})  [unwired: 1 in]
        n304 = Bundle(w25, w71) -> (w77:cluster{timestamp[], dbl[]})  [unwired: 1 in]
        n305 = Bundle(w25, w64) -> (w65:cluster{timestamp[], dbl[]})  [unwired: 1 in]
        n306 = Bundle(w25, w63) -> (w66:cluster{timestamp[], dbl[]})  [unwired: 1 in]
        n307 = Bundle(w25, w62) -> (w67:cluster{timestamp[], dbl[]})  [unwired: 1 in]
        n308 = Bundle(w25, w61) -> (w68:cluster{timestamp[], dbl[]})  [unwired: 1 in]
        n309 = Bundle(w25, w60) -> (w69:cluster{timestamp[], dbl[]})  [unwired: 1 in]
        n310 = Bundle(w25, w59) -> (w70:cluster{timestamp[], dbl[]})  [unwired: 1 in]
        n311 = Bundle(w25, w31) -> (w32:cluster{timestamp[], dbl[]})  [unwired: 1 in]
        n312 = Bundle(w25, w30) -> (w33:cluster{timestamp[], dbl[]})  [unwired: 1 in]
        n313 = Bundle(w25, w29) -> (w34:cluster{timestamp[], dbl[]})  [unwired: 1 in]
        n314 = Bundle(w25, w28) -> (w35:cluster{timestamp[], dbl[]})  [unwired: 1 in]
        n315 = Bundle(w25, w27) -> (w36:cluster{timestamp[], dbl[]})  [unwired: 1 in]
        n316 = Bundle(w25, w26) -> (w37:cluster{timestamp[], dbl[]})  [unwired: 1 in]
        n317 = Bundle(w25, w24) -> (w43:cluster{timestamp[], dbl[]})  [unwired: 1 in]
        n318 = Bundle(w25, w23) -> (w42:cluster{timestamp[], dbl[]})  [unwired: 1 in]
        n319 = Bundle(w25, w22) -> (w41:cluster{timestamp[], dbl[]})  [unwired: 1 in]
        n320 = Bundle(w25, w21) -> (w40:cluster{timestamp[], dbl[]})  [unwired: 1 in]
        n321 = Bundle(w25, w20) -> (w39:cluster{timestamp[], dbl[]})  [unwired: 1 in]
        n322 = Bundle(w25, w19) -> (w38:cluster{timestamp[], dbl[]})  [unwired: 1 in]
        n323 = Bundle(w25, w18) -> (w44:cluster{timestamp[], dbl[]})  [unwired: 1 in]
        n324 = Bundle(w25, w17) -> (w45:cluster{timestamp[], dbl[]})  [unwired: 1 in]
        n325 = Bundle(w25, w16) -> (w46:cluster{timestamp[], dbl[]})  [unwired: 1 in]
        n326 = Bundle(w25, w15) -> (w47:cluster{timestamp[], dbl[]})  [unwired: 1 in]
        n327 = Bundle(w25, w14) -> (w48:cluster{timestamp[], dbl[]})  [unwired: 1 in]
        n328 = Bundle(w25, w13) -> (w49:cluster{timestamp[], dbl[]})  [unwired: 1 in]
        n329 = Bundle(w25, w12) -> (w55:cluster{timestamp[], dbl[]})  [unwired: 1 in]
        n330 = Bundle(w25, w11) -> (w54:cluster{timestamp[], dbl[]})  [unwired: 1 in]
        n331 = Bundle(w25, w10) -> (w53:cluster{timestamp[], dbl[]})  [unwired: 1 in]
        n332 = Bundle(w25, w9) -> (w52:cluster{timestamp[], dbl[]})  [unwired: 1 in]
        n333 = Bundle(w25, w8) -> (w51:cluster{timestamp[], dbl[]})  [unwired: 1 in]
        n334 = Bundle(w25, w7) -> (w50:cluster{timestamp[], dbl[]})  [unwired: 1 in]
        n335 = Array Size(array=w25) -> (size(s)=w687:i32)
        n336 = Decrement(x=w687) -> (x-1=w688:i32)
        n337 = Build Array(w108, w107, w106, w105, w104, w103) -> (w102:cluster{timestamp[], dbl[]}[])
        "L1-Current_Full" <- w102
        "L1-Current_Zoomed" <- w102
        n338 = Build Array(w89, w90, w91, w92, w93, w94) -> (w58:cluster{timestamp[], dbl[]}[])
        "L2-Current_Full" <- w58
        "L2-Current_Zoomed" <- w58
        n339 = Build Array(w82, w81, w80, w79, w78, w77) -> (w57:cluster{timestamp[], dbl[]}[])
        "L3-Current_Full" <- w57
        "L3-Current_Zoomed" <- w57
        n340 = Build Array(w65, w66, w67, w68, w69, w70) -> (w56:cluster{timestamp[], dbl[]}[])
        "L4-Current_Zoomed" <- w56
        "L4-Current_Full" <- w56
        n341 = Build Array(w32, w33, w34, w35, w36, w37) -> (→"L1-Voltage":cluster{timestamp[], dbl[]}[])
        n342 = Build Array(w43, w42, w41, w40, w39, w38) -> (→"L2-Voltage":cluster{timestamp[], dbl[]}[])
        n343 = Build Array(w44, w45, w46, w47, w48, w49) -> (→"L3-Voltage":cluster{timestamp[], dbl[]}[])
        n344 = Build Array(w55, w54, w53, w52, w51, w50) -> (→"L4-Voltage":cluster{timestamp[], dbl[]}[])
        n345 = Index Array(array=w25, index=w688) -> (element=w686:timestamp)
        n346 = Index Array(array=w25, index=0) -> (element=w689:timestamp)
        n347 = Subtract(x=w686, y=w689) -> (x-y=w690:dbl)
        n348 = Divide(x=w690, y=60.0) -> (x/y=w691:dbl)
        n349 = Divide(x=w691, y="Window size [min]") -> (x/y=w692:dbl)
        n350 = Round Toward -Infinity(1:w692) -> (0:w439:dbl)
        n351 = for {
          tunnel: w25 -> [_] mode=indexing
          tunnel: [w1174] -> w101 mode=indexing
          tunnel: "Threshold [uA]" -> [w1174]
        }
        n352 = Decrement(x=w439) -> (x-1=w438:dbl)
        n353 = Bundle(w25, w101) -> (w646:cluster{timestamp[], dbl[]})  [unwired: 1 in]
        n354 = for {
          N: w438 -> [w1274]
          tunnel: w59 -> [w1311]
          tunnel: w25 -> [w1309]
          tunnel: "Window size [min]" -> [w1211]
          tunnel: [w1310] -> w477 mode=indexing
          tunnel: [w1301] -> w465 mode=indexing
          shift-right: [w1306] -> w462
          shift-left: w683 -> [w1304]
          tunnel: [w1300] -> w360 mode=indexing
          shift-right: [w1302] -> _
          shift-left: w683 -> [w1303]
          tunnel: "Threshold [uA]" -> [w1212]
          tunnel: w60 -> [w1299]
          tunnel: w61 -> [w1298]
          tunnel: w62 -> [w1297]
          tunnel: w63 -> [w1296]
          tunnel: w64 -> [w1295]
          tunnel: [w1294] -> w361 mode=indexing
          tunnel: [w1293] -> w466 mode=indexing
          tunnel: [w1292] -> w467 mode=indexing
          tunnel: [w1291] -> w362 mode=indexing
          tunnel: [w1290] -> w468 mode=indexing
          tunnel: [w1289] -> w363 mode=indexing
          tunnel: [w1288] -> w469 mode=indexing
          tunnel: [w1287] -> w364 mode=indexing
          tunnel: [w1286] -> w365 mode=indexing
          tunnel: [w1285] -> w470 mode=indexing
          tunnel: [w1262] -> w526 mode=indexing
          tunnel: [w1263] -> w366 mode=indexing
          tunnel: [w1264] -> w367 mode=indexing
          tunnel: [w1265] -> w527 mode=indexing
          tunnel: [w1266] -> w528 mode=indexing
          tunnel: [w1267] -> w368 mode=indexing
          tunnel: [w1268] -> w529 mode=indexing
          tunnel: [w1269] -> w530 mode=indexing
          tunnel: [w1270] -> w370 mode=indexing
          tunnel: [w1271] -> w371 mode=indexing
          tunnel: [w1272] -> w531 mode=indexing
          tunnel: [w1261] -> w369 mode=indexing
          tunnel: w71 -> [w1259]
          tunnel: w72 -> [w1258]
          tunnel: w73 -> [w1257]
          tunnel: w74 -> [w1256]
          tunnel: w75 -> [w1255]
          tunnel: w76 -> [w1254]
          tunnel: w83 -> [w1253]
          tunnel: w84 -> [w1252]
          tunnel: w85 -> [w1251]
          tunnel: w86 -> [w1250]
          tunnel: w87 -> [w1249]
          tunnel: w88 -> [w1248]
          tunnel: w95 -> [w1247]
          tunnel: w96 -> [w1246]
          tunnel: w97 -> [w1245]
          tunnel: w98 -> [w1244]
          tunnel: w99 -> [w1243]
          tunnel: w100 -> [w1242]
          tunnel: [w1213] -> w580 mode=indexing
          tunnel: [w1214] -> w426 mode=indexing
          tunnel: [w1215] -> w427 mode=indexing
          tunnel: [w1216] -> w581 mode=indexing
          tunnel: [w1217] -> w582 mode=indexing
          tunnel: [w1218] -> w428 mode=indexing
          tunnel: [w1219] -> w583 mode=indexing
          tunnel: [w1220] -> w429 mode=indexing
          tunnel: [w1221] -> w584 mode=indexing
          tunnel: [w1222] -> w430 mode=indexing
          tunnel: [w1223] -> w431 mode=indexing
          tunnel: [w1224] -> w585 mode=indexing
          tunnel: [w1235] -> w670 mode=indexing
          tunnel: [w1234] -> w432 mode=indexing
          tunnel: [w1233] -> w433 mode=indexing
          tunnel: [w1232] -> w669 mode=indexing
          tunnel: [w1231] -> w668 mode=indexing
          tunnel: [w1230] -> w434 mode=indexing
          tunnel: [w1229] -> w667 mode=indexing
          tunnel: [w1228] -> w666 mode=indexing
          tunnel: [w1227] -> w436 mode=indexing
          tunnel: [w1226] -> w437 mode=indexing
          tunnel: [w1225] -> w665 mode=indexing
          tunnel: [w1236] -> w435 mode=indexing
          tunnel: [w1199] -> w647 mode=indexing
          tunnel: [w1198] -> w648 mode=indexing
          tunnel: [w1197] -> w649 mode=indexing
          tunnel: [w1196] -> w650 mode=indexing
          tunnel: [w1195] -> w651 mode=indexing
          tunnel: [w1194] -> w652 mode=indexing
          tunnel: [w1193] -> w579 mode=indexing
          tunnel: [w1192] -> w578 mode=indexing
          tunnel: [w1191] -> w577 mode=indexing
          tunnel: [w1190] -> w576 mode=indexing
          tunnel: [w1189] -> w575 mode=indexing
          tunnel: [w1188] -> w574 mode=indexing
          tunnel: [w1187] -> w525 mode=indexing
          tunnel: [w1186] -> w524 mode=indexing
          tunnel: [w1185] -> w523 mode=indexing
          tunnel: [w1184] -> w522 mode=indexing
          tunnel: [w1183] -> w521 mode=indexing
          tunnel: [w1182] -> w520 mode=indexing
          tunnel: [w1181] -> w476 mode=indexing
          tunnel: [w1180] -> w475 mode=indexing
          tunnel: [w1179] -> w474 mode=indexing
          tunnel: [w1178] -> w473 mode=indexing
          tunnel: [w1177] -> w472 mode=indexing
          tunnel: [w1176] -> w471 mode=indexing
          i -> [w1278]
          n355 = Decrement(x=w1274) -> (x-1=w1273:i32)
          n356 = while {
            tunnel: w1311 -> [w1374]
            tunnel: w1309 -> [w1373]
            tunnel: [w1371] -> w1279 mode=indexing
            tunnel: w1211 -> [w1368]
            tunnel: w1303 -> [w1364]
            tunnel: [w1346] -> w1302
            tunnel: [w1361] -> w1305
            tunnel: [w1360] -> w1307
            tunnel: [w1358] -> w1284 mode=indexing
            tunnel: w1299 -> [w1357]
            tunnel: w1298 -> [w1356]
            tunnel: w1297 -> [w1355]
            tunnel: w1296 -> [w1354]
            tunnel: w1295 -> [w1353]
            tunnel: [w1352] -> w1283 mode=indexing
            tunnel: [w1351] -> w1282 mode=indexing
            tunnel: [w1350] -> w1281 mode=indexing
            tunnel: [w1349] -> w1280 mode=indexing
            tunnel: [w1348] -> w1260 mode=indexing
            tunnel: [w1347] -> w1241 mode=indexing
            tunnel: [w1345] -> w1240 mode=indexing
            tunnel: [w1344] -> w1239 mode=indexing
            tunnel: [w1343] -> w1238 mode=indexing
            tunnel: [w1342] -> w1237 mode=indexing
            tunnel: [w1341] -> w1210 mode=indexing
            tunnel: [w1340] -> w1209 mode=indexing
            tunnel: [w1339] -> w1208 mode=indexing
            tunnel: [w1338] -> w1207 mode=indexing
            tunnel: [w1337] -> w1206 mode=indexing
            tunnel: [w1336] -> w1205 mode=indexing
            tunnel: [w1335] -> w1204 mode=indexing
            tunnel: [w1334] -> w1203 mode=indexing
            tunnel: [w1333] -> w1202 mode=indexing
            tunnel: [w1332] -> w1201 mode=indexing
            tunnel: [w1331] -> w1200 mode=indexing
            tunnel: [w1330] -> w1175 mode=indexing
            tunnel: w1259 -> [w1329]
            tunnel: w1258 -> [w1328]
            tunnel: w1257 -> [w1327]
            tunnel: w1256 -> [w1326]
            tunnel: w1255 -> [w1325]
            tunnel: w1254 -> [w1324]
            tunnel: w1253 -> [w1323]
            tunnel: w1252 -> [w1322]
            tunnel: w1251 -> [w1321]
            tunnel: w1250 -> [w1320]
            tunnel: w1248 -> [w1319]
            tunnel: w1249 -> [w1318]
            tunnel: w1247 -> [w1317]
            tunnel: w1246 -> [w1316]
            tunnel: w1245 -> [w1315]
            tunnel: w1244 -> [w1314]
            tunnel: w1243 -> [w1313]
            tunnel: w1242 -> [w1312]
            i -> [w1365]
            stop <- w1359 stop-if-true
            n357 = Add(x=w1365, y=w1364) -> (x+y=w1346:i32)
            n358 = Index Array(array=w1373, index=w1364) -> (element=w1369:timestamp)
            n359 = Index Array(array=w1312, index=w1346) -> (element=w1330:dbl)
            n360 = Index Array(array=w1313, index=w1346) -> (element=w1331:dbl)
            n361 = Index Array(array=w1314, index=w1346) -> (element=w1332:dbl)
            n362 = Index Array(array=w1315, index=w1346) -> (element=w1333:dbl)
            n363 = Index Array(array=w1316, index=w1346) -> (element=w1334:dbl)
            n364 = Index Array(array=w1317, index=w1346) -> (element=w1335:dbl)
            n365 = Index Array(array=w1319, index=w1346) -> (element=w1336:dbl)
            n366 = Index Array(array=w1318, index=w1346) -> (element=w1337:dbl)
            n367 = Index Array(array=w1320, index=w1346) -> (element=w1338:dbl)
            n368 = Index Array(array=w1321, index=w1346) -> (element=w1339:dbl)
            n369 = Index Array(array=w1322, index=w1346) -> (element=w1340:dbl)
            n370 = Index Array(array=w1323, index=w1346) -> (element=w1341:dbl)
            n371 = Index Array(array=w1324, index=w1346) -> (element=w1342:dbl)
            n372 = Index Array(array=w1325, index=w1346) -> (element=w1343:dbl)
            n373 = Index Array(array=w1326, index=w1346) -> (element=w1344:dbl)
            n374 = Index Array(array=w1327, index=w1346) -> (element=w1345:dbl)
            n375 = Index Array(array=w1328, index=w1346) -> (element=w1347:dbl)
            n376 = Index Array(array=w1329, index=w1346) -> (element=w1348:dbl)
            n377 = Index Array(array=w1353, index=w1346) -> (element=w1349:dbl)
            n378 = Index Array(array=w1354, index=w1346) -> (element=w1350:dbl)
            n379 = Index Array(array=w1355, index=w1346) -> (element=w1351:dbl)
            n380 = Index Array(array=w1356, index=w1346) -> (element=w1352:dbl)
            n381 = Index Array(array=w1357, index=w1346) -> (element=w1358:dbl)
            n382 = Index Array(array=w1374, index=w1346) -> (element=w1371:dbl)
            n383 = Index Array(array=w1373, index=w1346) -> (element=w1370:timestamp)
            n384 = Subtract(x=w1370, y=w1369) -> (x-y=w1363:dbl)
            n385 = Multiply(x=w1368, y=60.0) -> (x*y=w1362:dbl)
            n386 = Subtract(x=w1346, y=w1364) -> (x-y=w1360:i32)
            n387 = Greater Or Equal?(x=w1363, y=w1362) -> (x >= y?=w1359:bool)
            n388 = Divide(x=w1360, y=2) -> (x/y=w1367:dbl)
            n389 = Round To Nearest(number=w1367) -> (nearest integer value=w1361:dbl)
          }
          n390 = Divide(x=w1278, y=w1273) -> (x/y=w1277:dbl)
          n391 = Multiply(x=w1277, y=100.0) -> (x*y=→"Progress":dbl)
          n392 = Add(x=w1307, y=w1304) -> (x+y=w1306:i32)
          n393 = Add(x=w1305, y=w1304) -> (x+y=w1308:dbl)
          n394 = call "Window_Avg_and_Spark_Rate_Median.vi"("Window size [min]"=w1211, "Threshold"=w1212, "Current in"=w1175) -> ("Window Spark Rate"=w1226:dbl, "Window Avg"=w1225:dbl, "window median"=w1199:dbl)
          n395 = call "Window_Avg_and_Spark_Rate_Median.vi"("Window size [min]"=w1211, "Threshold"=w1212, "Current in"=w1200) -> ("Window Spark Rate"=w1227:dbl, "Window Avg"=w1228:dbl, "window median"=w1198:dbl)
          n396 = call "Window_Avg_and_Spark_Rate_Median.vi"("Window size [min]"=w1211, "Threshold"=w1212, "Current in"=w1201) -> ("Window Spark Rate"=w1236:dbl, "Window Avg"=w1229:dbl, "window median"=w1197:dbl)
          n397 = call "Window_Avg_and_Spark_Rate_Median.vi"("Window size [min]"=w1211, "Threshold"=w1212, "Current in"=w1202) -> ("Window Spark Rate"=w1230:dbl, "Window Avg"=w1231:dbl, "window median"=w1196:dbl)
          n398 = call "Window_Avg_and_Spark_Rate_Median.vi"("Window size [min]"=w1211, "Threshold"=w1212, "Current in"=w1203) -> ("Window Spark Rate"=w1233:dbl, "Window Avg"=w1232:dbl, "window median"=w1195:dbl)
          n399 = call "Window_Avg_and_Spark_Rate_Median.vi"("Window size [min]"=w1211, "Threshold"=w1212, "Current in"=w1204) -> ("Window Spark Rate"=w1234:dbl, "Window Avg"=w1235:dbl, "window median"=w1194:dbl)
          n400 = call "Window_Avg_and_Spark_Rate_Median.vi"("Window size [min]"=w1211, "Threshold"=w1212, "Current in"=w1205) -> ("Window Spark Rate"=w1223:dbl, "Window Avg"=w1224:dbl, "window median"=w1193:dbl)
          n401 = call "Window_Avg_and_Spark_Rate_Median.vi"("Window size [min]"=w1211, "Threshold"=w1212, "Current in"=w1206) -> ("Window Spark Rate"=w1222:dbl, "Window Avg"=w1221:dbl, "window median"=w1192:dbl)
          n402 = call "Window_Avg_and_Spark_Rate_Median.vi"("Window size [min]"=w1211, "Threshold"=w1212, "Current in"=w1207) -> ("Window Spark Rate"=w1220:dbl, "Window Avg"=w1219:dbl, "window median"=w1191:dbl)
          n403 = call "Window_Avg_and_Spark_Rate_Median.vi"("Window size [min]"=w1211, "Threshold"=w1212, "Current in"=w1208) -> ("Window Spark Rate"=w1218:dbl, "Window Avg"=w1217:dbl, "window median"=w1190:dbl)
          n404 = call "Window_Avg_and_Spark_Rate_Median.vi"("Window size [min]"=w1211, "Threshold"=w1212, "Current in"=w1209) -> ("Window Spark Rate"=w1215:dbl, "Window Avg"=w1216:dbl, "window median"=w1189:dbl)
          n405 = call "Window_Avg_and_Spark_Rate_Median.vi"("Window size [min]"=w1211, "Threshold"=w1212, "Current in"=w1210) -> ("Window Spark Rate"=w1214:dbl, "Window Avg"=w1213:dbl, "window median"=w1188:dbl)
          n406 = call "Window_Avg_and_Spark_Rate_Median.vi"("Window size [min]"=w1211, "Threshold"=w1212, "Current in"=w1237) -> ("Window Spark Rate"=w1271:dbl, "Window Avg"=w1272:dbl, "window median"=w1187:dbl)
          n407 = call "Window_Avg_and_Spark_Rate_Median.vi"("Window size [min]"=w1211, "Threshold"=w1212, "Current in"=w1238) -> ("Window Spark Rate"=w1270:dbl, "Window Avg"=w1269:dbl, "window median"=w1186:dbl)
          n408 = call "Window_Avg_and_Spark_Rate_Median.vi"("Window size [min]"=w1211, "Threshold"=w1212, "Current in"=w1239) -> ("Window Spark Rate"=w1261:dbl, "Window Avg"=w1268:dbl, "window median"=w1185:dbl)
          n409 = call "Window_Avg_and_Spark_Rate_Median.vi"("Window size [min]"=w1211, "Threshold"=w1212, "Current in"=w1240) -> ("Window Spark Rate"=w1267:dbl, "Window Avg"=w1266:dbl, "window median"=w1184:dbl)
          n410 = call "Window_Avg_and_Spark_Rate_Median.vi"("Window size [min]"=w1211, "Threshold"=w1212, "Current in"=w1241) -> ("Window Spark Rate"=w1264:dbl, "Window Avg"=w1265:dbl, "window median"=w1183:dbl)
          n411 = call "Window_Avg_and_Spark_Rate_Median.vi"("Window size [min]"=w1211, "Threshold"=w1212, "Current in"=w1260) -> ("Window Spark Rate"=w1263:dbl, "Window Avg"=w1262:dbl, "window median"=w1182:dbl)
          n412 = call "Window_Avg_and_Spark_Rate_Median.vi"("Window size [min]"=w1211, "Threshold"=w1212, "Current in"=w1280) -> ("Window Spark Rate"=w1286:dbl, "Window Avg"=w1285:dbl, "window median"=w1181:dbl)
          n413 = call "Window_Avg_and_Spark_Rate_Median.vi"("Window size [min]"=w1211, "Threshold"=w1212, "Current in"=w1281) -> ("Window Spark Rate"=w1287:dbl, "Window Avg"=w1288:dbl, "window median"=w1180:dbl)
          n414 = call "Window_Avg_and_Spark_Rate_Median.vi"("Window size [min]"=w1211, "Threshold"=w1212, "Current in"=w1282) -> ("Window Spark Rate"=w1289:dbl, "Window Avg"=w1290:dbl, "window median"=w1179:dbl)
          n415 = call "Window_Avg_and_Spark_Rate_Median.vi"("Window size [min]"=w1211, "Threshold"=w1212, "Current in"=w1283) -> ("Window Spark Rate"=w1291:dbl, "Window Avg"=w1292:dbl, "window median"=w1178:dbl)
          n416 = call "Window_Avg_and_Spark_Rate_Median.vi"("Window size [min]"=w1211, "Threshold"=w1212, "Current in"=w1284) -> ("Window Spark Rate"=w1294:dbl, "Window Avg"=w1293:dbl, "window median"=w1177:dbl)
          n417 = call "Window_Avg_and_Spark_Rate_Median.vi"("Window size [min]"=w1211, "Threshold"=w1212, "Current in"=w1279) -> ("Window Spark Rate"=w1300:dbl, "Window Avg"=w1301:dbl, "window median"=w1176:dbl)
          n418 = Index Array(array=w1309, index=w1308) -> (element=w1310:timestamp)
        }
        n419 = flat-sequence {
          tunnel: w646 -> [w697]
          tunnel: w102 -> [w696]
          tunnel: w58 -> [w695]
          tunnel: w57 -> [w694]
          tunnel: w56 -> [w693]
          frame #0 {
            # "Current Graphs"
            n420 = Build Array (concatenate)(w697, w696) -> (→"L1-Current [uA]":cluster{timestamp[], dbl[]}[])
            n421 = Build Array (concatenate)(w697, w695) -> (→"L2-Current [uA]":cluster{timestamp[], dbl[]}[])
            n422 = Build Array (concatenate)(w697, w694) -> (→"L3-Current [uA]":cluster{timestamp[], dbl[]}[])
            n423 = Build Array (concatenate)(w697, w693) -> (→"L4-Current [uA]":cluster{timestamp[], dbl[]}[])
          }
          frame #1 {
            n424 = property on="L1-Current_Full" class="XYGraph (strict)"() -> ("XScale.Maximum"=w704:dbl, "XScale.Minimum"=w705:dbl)  [unwired: 2 in, 2 out]
            n425 = property on="L1-Current_Full" class="XYGraph (strict)"() -> ("YScale.Maximum"=w706:dbl, "YScale.Minimum"=w707:dbl)  [unwired: 2 in, 2 out]
            n426 = property on="L3-Current_Full" class="XYGraph (strict)"() -> ("XScale.Maximum"=w723:dbl, "XScale.Minimum"=w722:dbl)  [unwired: 2 in, 2 out]
            n427 = property on="L3-Current_Full" class="XYGraph (strict)"() -> ("YScale.Maximum"=w721:dbl, "YScale.Minimum"=w720:dbl)  [unwired: 2 in, 2 out]
            n428 = property on="L1_Horizontal Slider" class="Slide (strict)"("Scale.Maximum"=w704, "Scale.Minimum"=w705) -> ()  [unwired: 2 in, 2 out]
            n429 = property on="L1_Vertical Slider" class="Slide (strict)"("Scale.Maximum"=w706, "Scale.Minimum"=w707) -> ()  [unwired: 2 in, 2 out]
            n430 = property on="L3_Horizontal Slider" class="Slide (strict)"("Scale.Maximum"=w723, "Scale.Minimum"=w722) -> ()  [unwired: 2 in, 2 out]
            n431 = property on="L3_Vertical Slider" class="Slide (strict)"("Scale.Maximum"=w721, "Scale.Minimum"=w720) -> ()  [unwired: 2 in, 2 out]
            n432 = property on="L1-Current_Zoomed" class="XYGraph (strict)"("XScale.Maximum"=w704, "XScale.Minimum"=w705) -> ()  [unwired: 2 in, 2 out]
            n433 = property on="L1-Current_Zoomed" class="XYGraph (strict)"("YScale.Maximum"=w706, "YScale.Minimum"=w707) -> ()  [unwired: 2 in, 2 out]
            n434 = property on="L3-Current_Zoomed" class="XYGraph (strict)"("XScale.Maximum"=w723, "XScale.Minimum"=w722) -> ()  [unwired: 2 in, 2 out]
            n435 = property on="L3-Current_Zoomed" class="XYGraph (strict)"("YScale.Maximum"=w721, "YScale.Minimum"=w720) -> ()  [unwired: 2 in, 2 out]
            n436 = Bundle("XScale.Maximum"=w704, "XScale.Minimum"=w705) -> (w703:T8)  [unwired: 1 in]
            n437 = Bundle("YScale.Maximum"=w706, "YScale.Minimum"=w707) -> (w702:T9)  [unwired: 1 in]
            n438 = Bundle("XScale.Maximum"=w723, "XScale.Minimum"=w722) -> (w724:T8)  [unwired: 1 in]
            n439 = Bundle("YScale.Maximum"=w721, "YScale.Minimum"=w720) -> (w725:T9)  [unwired: 1 in]
            n440 = property on="L1_Horizontal Slider" class="Slide (strict)"("Value"=w703) -> ()  [unwired: 2 in, 2 out]
            n441 = property on="L1_Vertical Slider" class="Slide (strict)"("Value"=w702) -> ()  [unwired: 2 in, 2 out]
            n442 = property on="L3_Horizontal Slider" class="Slide (strict)"("Value"=w724) -> ()  [unwired: 2 in, 2 out]
            n443 = property on="L3_Vertical Slider" class="Slide (strict)"("Value"=w725) -> ()  [unwired: 2 in, 2 out]
            n444 = property on="L2-Current_Full" class="XYGraph (strict)"() -> ("XScale.Maximum"=w711:dbl, "XScale.Minimum"=w710:dbl)  [unwired: 2 in, 2 out]
            n445 = property on="L2-Current_Full" class="XYGraph (strict)"() -> ("YScale.Maximum"=w709:dbl, "YScale.Minimum"=w708:dbl)  [unwired: 2 in, 2 out]
            n446 = property on="L4-Current_Full" class="XYGraph (strict)"() -> ("XScale.Maximum"=w716:dbl, "XScale.Minimum"=w717:dbl)  [unwired: 2 in, 2 out]
            n447 = property on="L4-Current_Full" class="XYGraph (strict)"() -> ("YScale.Maximum"=w718:dbl, "YScale.Minimum"=w719:dbl)  [unwired: 2 in, 2 out]
            n448 = property on="L2_Horizontal Slider" class="Slide (strict)"("Scale.Maximum"=w711, "Scale.Minimum"=w710) -> ()  [unwired: 2 in, 2 out]
            n449 = property on="L2_Vertical Slider" class="Slide (strict)"("Scale.Maximum"=w709, "Scale.Minimum"=w708) -> ()  [unwired: 2 in, 2 out]
            n450 = property on="L4_Horizontal Slider" class="Slide (strict)"("Scale.Maximum"=w716, "Scale.Minimum"=w717) -> ()  [unwired: 2 in, 2 out]
            n451 = property on="L4_Vertical Slider" class="Slide (strict)"("Scale.Maximum"=w718, "Scale.Minimum"=w719) -> ()  [unwired: 2 in, 2 out]
            n452 = property on="L2-Current_Zoomed" class="XYGraph (strict)"("XScale.Maximum"=w711, "XScale.Minimum"=w710) -> ()  [unwired: 2 in, 2 out]
            n453 = property on="L2-Current_Zoomed" class="XYGraph (strict)"("YScale.Maximum"=w709, "YScale.Minimum"=w708) -> ()  [unwired: 2 in, 2 out]
            n454 = property on="L4-Current_Zoomed" class="XYGraph (strict)"("XScale.Maximum"=w716, "XScale.Minimum"=w717) -> ()  [unwired: 2 in, 2 out]
            n455 = property on="L4-Current_Zoomed" class="XYGraph (strict)"("YScale.Maximum"=w718, "YScale.Minimum"=w719) -> ()  [unwired: 2 in, 2 out]
            n456 = Bundle("XScale.Maximum"=w711, "XScale.Minimum"=w710) -> (w712:T8)  [unwired: 1 in]
            n457 = Bundle("YScale.Maximum"=w709, "YScale.Minimum"=w708) -> (w713:T9)  [unwired: 1 in]
            n458 = Bundle("XScale.Maximum"=w716, "XScale.Minimum"=w717) -> (w715:T8)  [unwired: 1 in]
            n459 = Bundle("YScale.Maximum"=w718, "YScale.Minimum"=w719) -> (w714:T9)  [unwired: 1 in]
            n460 = property on="L2_Horizontal Slider" class="Slide (strict)"("Value"=w712) -> ()  [unwired: 2 in, 2 out]
            n461 = property on="L2_Vertical Slider" class="Slide (strict)"("Value"=w713) -> ()  [unwired: 2 in, 2 out]
            n462 = property on="L4_Horizontal Slider" class="Slide (strict)"("Value"=w715) -> ()  [unwired: 2 in, 2 out]
            n463 = property on="L4_Vertical Slider" class="Slide (strict)"("Value"=w714) -> ()  [unwired: 2 in, 2 out]
          }
        }
        n464 = call "Statistic_tail_forming.vi"("Spark/min_IN"=w437) -> ("Spark/min_OUT"=w425:dbl[])
        n465 = call "Statistic_tail_forming.vi"("Spark/min_IN"=w436) -> ("Spark/min_OUT"=w423:dbl[])
        n466 = call "Statistic_tail_forming.vi"("Spark/min_IN"=w435) -> ("Spark/min_OUT"=w422:dbl[])
        n467 = call "Statistic_tail_forming.vi"("Spark/min_IN"=w434) -> ("Spark/min_OUT"=w421:dbl[])
        n468 = call "Statistic_tail_forming.vi"("Spark/min_IN"=w433) -> ("Spark/min_OUT"=w420:dbl[])
        n469 = call "Statistic_tail_forming.vi"("Spark/min_IN"=w432) -> ("Spark/min_OUT"=w419:dbl[])
        n470 = call "Statistic_tail_forming.vi"("Spark/min_IN"=w431) -> ("Spark/min_OUT"=w418:dbl[])
        n471 = call "Statistic_tail_forming.vi"("Spark/min_IN"=w430) -> ("Spark/min_OUT"=w417:dbl[])
        n472 = call "Statistic_tail_forming.vi"("Spark/min_IN"=w429) -> ("Spark/min_OUT"=w416:dbl[])
        n473 = call "Statistic_tail_forming.vi"("Spark/min_IN"=w428) -> ("Spark/min_OUT"=w415:dbl[])
        n474 = call "Statistic_tail_forming.vi"("Spark/min_IN"=w427) -> ("Spark/min_OUT"=w414:dbl[])
        n475 = call "Statistic_tail_forming.vi"("Spark/min_IN"=w426) -> ("Spark/min_OUT"=w413:dbl[])
        n476 = call <vilib>:"General Histogram.vi"("X"=w425, "max"=w411, "min"=w410, "# bins"=w412) -> ("Histogram Graph"=w424:T10)  [unwired: 7 in, 4 out]
        n477 = call <vilib>:"General Histogram.vi"("X"=w423, "max"=w411, "min"=w410, "# bins"=w412) -> ("Histogram Graph"=w409:T10)  [unwired: 7 in, 4 out]
        n478 = call <vilib>:"General Histogram.vi"("X"=w422, "max"=w411, "min"=w410, "# bins"=w412) -> ("Histogram Graph"=w408:T10)  [unwired: 7 in, 4 out]
        n479 = call <vilib>:"General Histogram.vi"("X"=w421, "max"=w411, "min"=w410, "# bins"=w412) -> ("Histogram Graph"=w407:T10)  [unwired: 7 in, 4 out]
        n480 = call <vilib>:"General Histogram.vi"("X"=w420, "max"=w411, "min"=w410, "# bins"=w412) -> ("Histogram Graph"=w406:T10)  [unwired: 7 in, 4 out]
        n481 = call <vilib>:"General Histogram.vi"("X"=w419, "max"=w411, "min"=w410, "# bins"=w412) -> ("Histogram Graph"=w405:T10)  [unwired: 7 in, 4 out]
        n482 = call <vilib>:"General Histogram.vi"("X"=w418, "max"=w411, "min"=w410, "# bins"=w412) -> ("Histogram Graph"=w404:T10)  [unwired: 7 in, 4 out]
        n483 = call <vilib>:"General Histogram.vi"("X"=w417, "max"=w411, "min"=w410, "# bins"=w412) -> ("Histogram Graph"=w403:T10)  [unwired: 7 in, 4 out]
        n484 = call <vilib>:"General Histogram.vi"("X"=w416, "max"=w411, "min"=w410, "# bins"=w412) -> ("Histogram Graph"=w402:T10)  [unwired: 7 in, 4 out]
        n485 = call <vilib>:"General Histogram.vi"("X"=w415, "max"=w411, "min"=w410, "# bins"=w412) -> ("Histogram Graph"=w401:T10)  [unwired: 7 in, 4 out]
        n486 = call <vilib>:"General Histogram.vi"("X"=w414, "max"=w411, "min"=w410, "# bins"=w412) -> ("Histogram Graph"=w400:T10)  [unwired: 7 in, 4 out]
        n487 = call <vilib>:"General Histogram.vi"("X"=w413, "max"=w411, "min"=w410, "# bins"=w412) -> ("Histogram Graph"=w399:T10)  [unwired: 7 in, 4 out]
        n488 = Build Array(w424, w409, w408, w407, w406, w405) -> (→"Spark-rate statistic_L1":T5)
        n489 = Build Array(w404, w403, w402, w401, w400, w399) -> (→"Spark-rate statistic_L2":T5)
        n490 = call "Statistic_tail_forming.vi"("Spark/min_IN"=w371) -> ("Spark/min_OUT"=w372:dbl[])
        n491 = call "Statistic_tail_forming.vi"("Spark/min_IN"=w370) -> ("Spark/min_OUT"=w374:dbl[])
        n492 = call "Statistic_tail_forming.vi"("Spark/min_IN"=w369) -> ("Spark/min_OUT"=w375:dbl[])
        n493 = call "Statistic_tail_forming.vi"("Spark/min_IN"=w368) -> ("Spark/min_OUT"=w376:dbl[])
        n494 = call "Statistic_tail_forming.vi"("Spark/min_IN"=w367) -> ("Spark/min_OUT"=w377:dbl[])
        n495 = call "Statistic_tail_forming.vi"("Spark/min_IN"=w366) -> ("Spark/min_OUT"=w378:dbl[])
        n496 = call "Statistic_tail_forming.vi"("Spark/min_IN"=w365) -> ("Spark/min_OUT"=w379:dbl[])
        n497 = call "Statistic_tail_forming.vi"("Spark/min_IN"=w364) -> ("Spark/min_OUT"=w380:dbl[])
        n498 = call "Statistic_tail_forming.vi"("Spark/min_IN"=w363) -> ("Spark/min_OUT"=w381:dbl[])
        n499 = call "Statistic_tail_forming.vi"("Spark/min_IN"=w362) -> ("Spark/min_OUT"=w382:dbl[])
        n500 = call "Statistic_tail_forming.vi"("Spark/min_IN"=w361) -> ("Spark/min_OUT"=w383:dbl[])
        n501 = call "Statistic_tail_forming.vi"("Spark/min_IN"=w360) -> ("Spark/min_OUT"=w384:dbl[])
        n502 = call "Last_Window.vi"("Produced_Time"=w477, "Windows_Last_Index"=w462, "Window_Spark_Rate_IN"=w437, "Threshold [uA]"="Threshold [uA]", "Window_Median_IN"=w647, "Window_Avg_IN"=w665, "Window size [min]"="Window size [min]", "Origin_Time"=w25, "Origin_Current_IN"=w100) -> ("Time_Out"=w664:timestamp[], "Window_Avg_OUT"=w680:dbl[], "Window_Median_OUT"=w663:dbl[], "Window_Spark_Rate_OUT"=w681:dbl[])  [unwired: 2 in, 1 out]
        n503 = call "Last_Window.vi"("Produced_Time"=w477, "Windows_Last_Index"=w462, "Window_Spark_Rate_IN"=w436, "Threshold [uA]"="Threshold [uA]", "Window_Median_IN"=w648, "Window_Avg_IN"=w666, "Window size [min]"="Window size [min]", "Origin_Time"=w25, "Origin_Current_IN"=w99) -> ("Time_Out"=w662:timestamp[], "Window_Avg_OUT"=w676:dbl[], "Window_Median_OUT"=w661:dbl[], "Window_Spark_Rate_OUT"=w677:dbl[])  [unwired: 2 in, 1 out]
        n504 = call "Last_Window.vi"("Produced_Time"=w477, "Windows_Last_Index"=w462, "Window_Spark_Rate_IN"=w435, "Threshold [uA]"="Threshold [uA]", "Window_Median_IN"=w649, "Window_Avg_IN"=w667, "Window size [min]"="Window size [min]", "Origin_Time"=w25, "Origin_Current_IN"=w98) -> ("Time_Out"=w659:timestamp[], "Window_Avg_OUT"=w679:dbl[], "Window_Median_OUT"=w660:dbl[], "Window_Spark_Rate_OUT"=w678:dbl[])  [unwired: 2 in, 1 out]
        n505 = call "Last_Window.vi"("Produced_Time"=w477, "Windows_Last_Index"=w462, "Window_Spark_Rate_IN"=w434, "Threshold [uA]"="Threshold [uA]", "Window_Median_IN"=w650, "Window_Avg_IN"=w668, "Window size [min]"="Window size [min]", "Origin_Time"=w25, "Origin_Current_IN"=w97) -> ("Time_Out"=w658:timestamp[], "Window_Avg_OUT"=w674:dbl[], "Window_Median_OUT"=w657:dbl[], "Window_Spark_Rate_OUT"=w675:dbl[])  [unwired: 2 in, 1 out]
        n506 = call "Last_Window.vi"("Produced_Time"=w477, "Windows_Last_Index"=w462, "Window_Spark_Rate_IN"=w433, "Threshold [uA]"="Threshold [uA]", "Window_Median_IN"=w651, "Window_Avg_IN"=w669, "Window size [min]"="Window size [min]", "Origin_Time"=w25, "Origin_Current_IN"=w96) -> ("Time_Out"=w656:timestamp[], "Window_Avg_OUT"=w672:dbl[], "Window_Median_OUT"=w655:dbl[], "Window_Spark_Rate_OUT"=w673:dbl[])  [unwired: 2 in, 1 out]
        n507 = call "Last_Window.vi"("Produced_Time"=w477, "Windows_Last_Index"=w462, "Window_Spark_Rate_IN"=w432, "Threshold [uA]"="Threshold [uA]", "Window_Median_IN"=w652, "Window_Avg_IN"=w670, "Window size [min]"="Window size [min]", "Origin_Time"=w25, "Origin_Current_IN"=w95) -> ("Time_Out"=w654:timestamp[], "Window_Avg_OUT"=w682:dbl[], "Window_Median_OUT"=w653:dbl[], "Window_Spark_Rate_OUT"=w671:dbl[])  [unwired: 2 in, 1 out]
        n508 = call "Last_Window.vi"("Produced_Time"=w477, "Windows_Last_Index"=w462, "Window_Spark_Rate_IN"=w431, "Threshold [uA]"="Threshold [uA]", "Window_Median_IN"=w579, "Window_Avg_IN"=w585, "Window size [min]"="Window size [min]", "Origin_Time"=w25, "Origin_Current_IN"=w88) -> ("Time_Out"=w598:timestamp[], "Window_Avg_OUT"=w588:dbl[], "Window_Median_OUT"=w599:dbl[], "Window_Spark_Rate_OUT"=w587:dbl[])  [unwired: 2 in, 1 out]
        n509 = call "Last_Window.vi"("Produced_Time"=w477, "Windows_Last_Index"=w462, "Window_Spark_Rate_IN"=w430, "Threshold [uA]"="Threshold [uA]", "Window_Median_IN"=w578, "Window_Avg_IN"=w584, "Window size [min]"="Window size [min]", "Origin_Time"=w25, "Origin_Current_IN"=w87) -> ("Time_Out"=w600:timestamp[], "Window_Avg_OUT"=w592:dbl[], "Window_Median_OUT"=w601:dbl[], "Window_Spark_Rate_OUT"=w591:dbl[])  [unwired: 2 in, 1 out]
        n510 = call "Last_Window.vi"("Produced_Time"=w477, "Windows_Last_Index"=w462, "Window_Spark_Rate_IN"=w429, "Threshold [uA]"="Threshold [uA]", "Window_Median_IN"=w577, "Window_Avg_IN"=w583, "Window size [min]"="Window size [min]", "Origin_Time"=w25, "Origin_Current_IN"=w86) -> ("Time_Out"=w603:timestamp[], "Window_Avg_OUT"=w589:dbl[], "Window_Median_OUT"=w602:dbl[], "Window_Spark_Rate_OUT"=w590:dbl[])  [unwired: 2 in, 1 out]
        n511 = call "Last_Window.vi"("Produced_Time"=w477, "Windows_Last_Index"=w462, "Window_Spark_Rate_IN"=w428, "Threshold [uA]"="Threshold [uA]", "Window_Median_IN"=w576, "Window_Avg_IN"=w582, "Window size [min]"="Window size [min]", "Origin_Time"=w25, "Origin_Current_IN"=w85) -> ("Time_Out"=w604:timestamp[], "Window_Avg_OUT"=w594:dbl[], "Window_Median_OUT"=w605:dbl[], "Window_Spark_Rate_OUT"=w593:dbl[])  [unwired: 2 in, 1 out]
        n512 = call "Last_Window.vi"("Produced_Time"=w477, "Windows_Last_Index"=w462, "Window_Spark_Rate_IN"=w427, "Threshold [uA]"="Threshold [uA]", "Window_Median_IN"=w575, "Window_Avg_IN"=w581, "Window size [min]"="Window size [min]", "Origin_Time"=w25, "Origin_Current_IN"=w84) -> ("Time_Out"=w606:timestamp[], "Window_Avg_OUT"=w596:dbl[], "Window_Median_OUT"=w607:dbl[], "Window_Spark_Rate_OUT"=w595:dbl[])  [unwired: 2 in, 1 out]
        n513 = call "Last_Window.vi"("Produced_Time"=w477, "Windows_Last_Index"=w462, "Window_Spark_Rate_IN"=w426, "Threshold [uA]"="Threshold [uA]", "Window_Median_IN"=w574, "Window_Avg_IN"=w580, "Window size [min]"="Window size [min]", "Origin_Time"=w25, "Origin_Current_IN"=w83) -> ("Time_Out"=w608:timestamp[], "Window_Avg_OUT"=w586:dbl[], "Window_Median_OUT"=w609:dbl[], "Window_Spark_Rate_OUT"=w597:dbl[])  [unwired: 2 in, 1 out]
        n514 = call "Last_Window.vi"("Produced_Time"=w477, "Windows_Last_Index"=w462, "Window_Spark_Rate_IN"=w371, "Threshold [uA]"="Threshold [uA]", "Window_Median_IN"=w525, "Window_Avg_IN"=w531, "Window size [min]"="Window size [min]", "Origin_Time"=w25, "Origin_Current_IN"=w76) -> ("Time_Out"=w561:timestamp[], "Window_Avg_OUT"=w571:dbl[], "Window_Median_OUT"=w560:dbl[], "Window_Spark_Rate_OUT"=w572:dbl[])  [unwired: 2 in, 1 out]
        n515 = call "Last_Window.vi"("Produced_Time"=w477, "Windows_Last_Index"=w462, "Window_Spark_Rate_IN"=w370, "Threshold [uA]"="Threshold [uA]", "Window_Median_IN"=w524, "Window_Avg_IN"=w530, "Window size [min]"="Window size [min]", "Origin_Time"=w25, "Origin_Current_IN"=w75) -> ("Time_Out"=w559:timestamp[], "Window_Avg_OUT"=w567:dbl[], "Window_Median_OUT"=w558:dbl[], "Window_Spark_Rate_OUT"=w568:dbl[])  [unwired: 2 in, 1 out]
        n516 = call "Last_Window.vi"("Produced_Time"=w477, "Windows_Last_Index"=w462, "Window_Spark_Rate_IN"=w369, "Threshold [uA]"="Threshold [uA]", "Window_Median_IN"=w523, "Window_Avg_IN"=w529, "Window size [min]"="Window size [min]", "Origin_Time"=w25, "Origin_Current_IN"=w74) -> ("Time_Out"=w556:timestamp[], "Window_Avg_OUT"=w570:dbl[], "Window_Median_OUT"=w557:dbl[], "Window_Spark_Rate_OUT"=w569:dbl[])  [unwired: 2 in, 1 out]
        n517 = call "Last_Window.vi"("Produced_Time"=w477, "Windows_Last_Index"=w462, "Window_Spark_Rate_IN"=w368, "Threshold [uA]"="Threshold [uA]", "Window_Median_IN"=w522, "Window_Avg_IN"=w528, "Window size [min]"="Window size [min]", "Origin_Time"=w25, "Origin_Current_IN"=w73) -> ("Time_Out"=w555:timestamp[], "Window_Avg_OUT"=w565:dbl[], "Window_Median_OUT"=w554:dbl[], "Window_Spark_Rate_OUT"=w566:dbl[])  [unwired: 2 in, 1 out]
        n518 = call "Last_Window.vi"("Produced_Time"=w477, "Windows_Last_Index"=w462, "Window_Spark_Rate_IN"=w367, "Threshold [uA]"="Threshold [uA]", "Window_Median_IN"=w521, "Window_Avg_IN"=w527, "Window size [min]"="Window size [min]", "Origin_Time"=w25, "Origin_Current_IN"=w72) -> ("Time_Out"=w553:timestamp[], "Window_Avg_OUT"=w563:dbl[], "Window_Median_OUT"=w552:dbl[], "Window_Spark_Rate_OUT"=w564:dbl[])  [unwired: 2 in, 1 out]
        n519 = call "Last_Window.vi"("Produced_Time"=w477, "Windows_Last_Index"=w462, "Window_Spark_Rate_IN"=w366, "Threshold [uA]"="Threshold [uA]", "Window_Median_IN"=w520, "Window_Avg_IN"=w526, "Window size [min]"="Window size [min]", "Origin_Time"=w25, "Origin_Current_IN"=w71) -> ("Time_Out"=w551:timestamp[], "Window_Avg_OUT"=w573:dbl[], "Window_Median_OUT"=w550:dbl[], "Window_Spark_Rate_OUT"=w562:dbl[])  [unwired: 2 in, 1 out]
        n520 = call "Last_Window.vi"("Produced_Time"=w477, "Windows_Last_Index"=w462, "Window_Spark_Rate_IN"=w365, "Threshold [uA]"="Threshold [uA]", "Window_Median_IN"=w476, "Window_Avg_IN"=w470, "Window size [min]"="Window size [min]", "Origin_Time"=w25, "Origin_Current_IN"=w64) -> ("Time_Out"=w490:timestamp[], "Window_Avg_OUT"=w480:dbl[], "Window_Median_OUT"=w491:dbl[], "Window_Spark_Rate_OUT"=w479:dbl[])  [unwired: 2 in, 1 out]
        n521 = call "Last_Window.vi"("Produced_Time"=w477, "Windows_Last_Index"=w462, "Window_Spark_Rate_IN"=w364, "Threshold [uA]"="Threshold [uA]", "Window_Median_IN"=w475, "Window_Avg_IN"=w469, "Window size [min]"="Window size [min]", "Origin_Time"=w25, "Origin_Current_IN"=w63) -> ("Time_Out"=w492:timestamp[], "Window_Avg_OUT"=w484:dbl[], "Window_Median_OUT"=w493:dbl[], "Window_Spark_Rate_OUT"=w483:dbl[])  [unwired: 2 in, 1 out]
        n522 = call "Last_Window.vi"("Produced_Time"=w477, "Windows_Last_Index"=w462, "Window_Spark_Rate_IN"=w363, "Threshold [uA]"="Threshold [uA]", "Window_Median_IN"=w474, "Window_Avg_IN"=w468, "Window size [min]"="Window size [min]", "Origin_Time"=w25, "Origin_Current_IN"=w62) -> ("Time_Out"=w495:timestamp[], "Window_Avg_OUT"=w481:dbl[], "Window_Median_OUT"=w494:dbl[], "Window_Spark_Rate_OUT"=w482:dbl[])  [unwired: 2 in, 1 out]
        n523 = call "Last_Window.vi"("Produced_Time"=w477, "Windows_Last_Index"=w462, "Window_Spark_Rate_IN"=w362, "Threshold [uA]"="Threshold [uA]", "Window_Median_IN"=w473, "Window_Avg_IN"=w467, "Window size [min]"="Window size [min]", "Origin_Time"=w25, "Origin_Current_IN"=w61) -> ("Time_Out"=w496:timestamp[], "Window_Avg_OUT"=w486:dbl[], "Window_Median_OUT"=w497:dbl[], "Window_Spark_Rate_OUT"=w485:dbl[])  [unwired: 2 in, 1 out]
        n524 = call "Last_Window.vi"("Produced_Time"=w477, "Windows_Last_Index"=w462, "Window_Spark_Rate_IN"=w361, "Threshold [uA]"="Threshold [uA]", "Window_Median_IN"=w472, "Window_Avg_IN"=w466, "Window size [min]"="Window size [min]", "Origin_Time"=w25, "Origin_Current_IN"=w60) -> ("Time_Out"=w498:timestamp[], "Window_Avg_OUT"=w488:dbl[], "Window_Median_OUT"=w499:dbl[], "Window_Spark_Rate_OUT"=w487:dbl[])  [unwired: 2 in, 1 out]
        n525 = call "Last_Window.vi"("Produced_Time"=w477, "Windows_Last_Index"=w462, "Window_Spark_Rate_IN"=w360, "Threshold [uA]"="Threshold [uA]", "Window_Median_IN"=w471, "Window_Avg_IN"=w465, "Window size [min]"="Window size [min]", "Origin_Time"=w25, "Origin_Current_IN"=w59) -> ("Time_Out"=w500:timestamp[], "Window_Avg_OUT"=w478:dbl[], "Window_Median_OUT"=w501:dbl[], "Window_Spark_Rate_OUT"=w489:dbl[])  [unwired: 2 in, 1 out]
        n526 = call <vilib>:"General Histogram.vi"("X"=w372, "max"=w386, "min"=w387, "# bins"=w385) -> ("Histogram Graph"=w373:T10)  [unwired: 7 in, 4 out]
        n527 = call <vilib>:"General Histogram.vi"("X"=w374, "max"=w386, "min"=w387, "# bins"=w385) -> ("Histogram Graph"=w388:T10)  [unwired: 7 in, 4 out]
        n528 = call <vilib>:"General Histogram.vi"("X"=w375, "max"=w386, "min"=w387, "# bins"=w385) -> ("Histogram Graph"=w389:T10)  [unwired: 7 in, 4 out]
        n529 = call <vilib>:"General Histogram.vi"("X"=w376, "max"=w386, "min"=w387, "# bins"=w385) -> ("Histogram Graph"=w390:T10)  [unwired: 7 in, 4 out]
        n530 = call <vilib>:"General Histogram.vi"("X"=w377, "max"=w386, "min"=w387, "# bins"=w385) -> ("Histogram Graph"=w391:T10)  [unwired: 7 in, 4 out]
        n531 = call <vilib>:"General Histogram.vi"("X"=w378, "max"=w386, "min"=w387, "# bins"=w385) -> ("Histogram Graph"=w392:T10)  [unwired: 7 in, 4 out]
        n532 = call <vilib>:"General Histogram.vi"("X"=w379, "max"=w386, "min"=w387, "# bins"=w385) -> ("Histogram Graph"=w393:T10)  [unwired: 7 in, 4 out]
        n533 = call <vilib>:"General Histogram.vi"("X"=w380, "max"=w386, "min"=w387, "# bins"=w385) -> ("Histogram Graph"=w394:T10)  [unwired: 7 in, 4 out]
        n534 = call <vilib>:"General Histogram.vi"("X"=w381, "max"=w386, "min"=w387, "# bins"=w385) -> ("Histogram Graph"=w395:T10)  [unwired: 7 in, 4 out]
        n535 = call <vilib>:"General Histogram.vi"("X"=w382, "max"=w386, "min"=w387, "# bins"=w385) -> ("Histogram Graph"=w396:T10)  [unwired: 7 in, 4 out]
        n536 = call <vilib>:"General Histogram.vi"("X"=w383, "max"=w386, "min"=w387, "# bins"=w385) -> ("Histogram Graph"=w397:T10)  [unwired: 7 in, 4 out]
        n537 = call <vilib>:"General Histogram.vi"("X"=w384, "max"=w386, "min"=w387, "# bins"=w385) -> ("Histogram Graph"=w398:T10)  [unwired: 7 in, 4 out]
        n538 = Build Array(w373, w388, w389, w390, w391, w392) -> (→"Spark-rate statistic_L3":T5)
        n539 = Build Array(w393, w394, w395, w396, w397, w398) -> (→"Spark-rate statistic_L4":T5)
        n540 = Bundle("Time_Out"=w664, "Window_Avg_OUT"=w680) -> (w645:T11)  [unwired: 1 in]
        n541 = Bundle("Time_Out"=w664, "Window_Spark_Rate_OUT"=w681) -> (w639:T12)  [unwired: 1 in]
        n542 = Bundle("Time_Out"=w664, "Window_Median_OUT"=w663) -> (w633:T13)  [unwired: 1 in]
        n543 = Bundle("Time_Out"=w662, "Window_Avg_OUT"=w676) -> (w644:T11)  [unwired: 1 in]
        n544 = Bundle("Time_Out"=w662, "Window_Spark_Rate_OUT"=w677) -> (w638:T12)  [unwired: 1 in]
        n545 = Bundle("Time_Out"=w662, "Window_Median_OUT"=w661) -> (w632:T13)  [unwired: 1 in]
        n546 = Bundle("Time_Out"=w659, "Window_Avg_OUT"=w679) -> (w643:T11)  [unwired: 1 in]
        n547 = Bundle("Time_Out"=w659, "Window_Spark_Rate_OUT"=w678) -> (w637:T12)  [unwired: 1 in]
        n548 = Bundle("Time_Out"=w659, "Window_Median_OUT"=w660) -> (w631:T13)  [unwired: 1 in]
        n549 = Bundle("Time_Out"=w658, "Window_Avg_OUT"=w674) -> (w642:T11)  [unwired: 1 in]
        n550 = Bundle("Time_Out"=w658, "Window_Spark_Rate_OUT"=w675) -> (w636:T12)  [unwired: 1 in]
        n551 = Bundle("Time_Out"=w658, "Window_Median_OUT"=w657) -> (w630:T13)  [unwired: 1 in]
        n552 = Bundle("Time_Out"=w656, "Window_Avg_OUT"=w672) -> (w641:T11)  [unwired: 1 in]
        n553 = Bundle("Time_Out"=w656, "Window_Spark_Rate_OUT"=w673) -> (w635:T12)  [unwired: 1 in]
        n554 = Bundle("Time_Out"=w656, "Window_Median_OUT"=w655) -> (w629:T13)  [unwired: 1 in]
        n555 = Bundle("Time_Out"=w654, "Window_Avg_OUT"=w682) -> (w640:T11)  [unwired: 1 in]
        n556 = Bundle("Time_Out"=w654, "Window_Spark_Rate_OUT"=w671) -> (w634:T12)  [unwired: 1 in]
        n557 = Bundle("Time_Out"=w654, "Window_Median_OUT"=w653) -> (w628:T13)  [unwired: 1 in]
        n558 = Bundle("Time_Out"=w598, "Window_Avg_OUT"=w588) -> (w610:T11)  [unwired: 1 in]
        n559 = Bundle("Time_Out"=w598, "Window_Spark_Rate_OUT"=w587) -> (w616:T12)  [unwired: 1 in]
        n560 = Bundle("Time_Out"=w598, "Window_Median_OUT"=w599) -> (w622:T13)  [unwired: 1 in]
        n561 = Bundle("Time_Out"=w600, "Window_Avg_OUT"=w592) -> (w611:T11)  [unwired: 1 in]
        n562 = Bundle("Time_Out"=w600, "Window_Spark_Rate_OUT"=w591) -> (w617:T12)  [unwired: 1 in]
        n563 = Bundle("Time_Out"=w600, "Window_Median_OUT"=w601) -> (w623:T13)  [unwired: 1 in]
        n564 = Bundle("Time_Out"=w603, "Window_Avg_OUT"=w589) -> (w612:T11)  [unwired: 1 in]
        n565 = Bundle("Time_Out"=w603, "Window_Spark_Rate_OUT"=w590) -> (w618:T12)  [unwired: 1 in]
        n566 = Bundle("Time_Out"=w603, "Window_Median_OUT"=w602) -> (w624:T13)  [unwired: 1 in]
        n567 = Bundle("Time_Out"=w604, "Window_Avg_OUT"=w594) -> (w613:T11)  [unwired: 1 in]
        n568 = Bundle("Time_Out"=w604, "Window_Spark_Rate_OUT"=w593) -> (w619:T12)  [unwired: 1 in]
        n569 = Bundle("Time_Out"=w604, "Window_Median_OUT"=w605) -> (w625:T13)  [unwired: 1 in]
        n570 = Bundle("Time_Out"=w606, "Window_Avg_OUT"=w596) -> (w614:T11)  [unwired: 1 in]
        n571 = Bundle("Time_Out"=w606, "Window_Spark_Rate_OUT"=w595) -> (w620:T12)  [unwired: 1 in]
        n572 = Bundle("Time_Out"=w606, "Window_Median_OUT"=w607) -> (w626:T13)  [unwired: 1 in]
        n573 = Bundle("Time_Out"=w608, "Window_Avg_OUT"=w586) -> (w615:T11)  [unwired: 1 in]
        n574 = Bundle("Time_Out"=w608, "Window_Spark_Rate_OUT"=w597) -> (w621:T12)  [unwired: 1 in]
        n575 = Bundle("Time_Out"=w608, "Window_Median_OUT"=w609) -> (w627:T13)  [unwired: 1 in]
        n576 = Bundle("Time_Out"=w561, "Window_Avg_OUT"=w571) -> (w532:T11)  [unwired: 1 in]
        n577 = Bundle("Time_Out"=w561, "Window_Spark_Rate_OUT"=w572) -> (w544:T12)  [unwired: 1 in]
        n578 = Bundle("Time_Out"=w561, "Window_Median_OUT"=w560) -> (w538:T13)  [unwired: 1 in]
        n579 = Bundle("Time_Out"=w559, "Window_Avg_OUT"=w567) -> (w549:T11)  [unwired: 1 in]
        n580 = Bundle("Time_Out"=w559, "Window_Spark_Rate_OUT"=w568) -> (w543:T12)  [unwired: 1 in]
        n581 = Bundle("Time_Out"=w559, "Window_Median_OUT"=w558) -> (w537:T13)  [unwired: 1 in]
        n582 = Bundle("Time_Out"=w556, "Window_Avg_OUT"=w570) -> (w548:T11)  [unwired: 1 in]
        n583 = Bundle("Time_Out"=w556, "Window_Spark_Rate_OUT"=w569) -> (w542:T12)  [unwired: 1 in]
        n584 = Bundle("Time_Out"=w556, "Window_Median_OUT"=w557) -> (w536:T13)  [unwired: 1 in]
        n585 = Bundle("Time_Out"=w555, "Window_Avg_OUT"=w565) -> (w547:T11)  [unwired: 1 in]
        n586 = Bundle("Time_Out"=w555, "Window_Spark_Rate_OUT"=w566) -> (w541:T12)  [unwired: 1 in]
        n587 = Bundle("Time_Out"=w555, "Window_Median_OUT"=w554) -> (w535:T13)  [unwired: 1 in]
        n588 = Bundle("Time_Out"=w553, "Window_Avg_OUT"=w563) -> (w546:T11)  [unwired: 1 in]
        n589 = Bundle("Time_Out"=w553, "Window_Spark_Rate_OUT"=w564) -> (w540:T12)  [unwired: 1 in]
        n590 = Bundle("Time_Out"=w553, "Window_Median_OUT"=w552) -> (w534:T13)  [unwired: 1 in]
        n591 = Bundle("Time_Out"=w551, "Window_Avg_OUT"=w573) -> (w545:T11)  [unwired: 1 in]
        n592 = Bundle("Time_Out"=w551, "Window_Spark_Rate_OUT"=w562) -> (w539:T12)  [unwired: 1 in]
        n593 = Bundle("Time_Out"=w551, "Window_Median_OUT"=w550) -> (w533:T13)  [unwired: 1 in]
        n594 = Bundle("Time_Out"=w490, "Window_Avg_OUT"=w480) -> (w519:T11)  [unwired: 1 in]
        n595 = Bundle("Time_Out"=w490, "Window_Spark_Rate_OUT"=w479) -> (w507:T12)  [unwired: 1 in]
        n596 = Bundle("Time_Out"=w490, "Window_Median_OUT"=w491) -> (w513:T13)  [unwired: 1 in]
        n597 = Bundle("Time_Out"=w492, "Window_Avg_OUT"=w484) -> (w502:T11)  [unwired: 1 in]
        n598 = Bundle("Time_Out"=w492, "Window_Spark_Rate_OUT"=w483) -> (w508:T12)  [unwired: 1 in]
        n599 = Bundle("Time_Out"=w492, "Window_Median_OUT"=w493) -> (w514:T13)  [unwired: 1 in]
        n600 = Bundle("Time_Out"=w495, "Window_Avg_OUT"=w481) -> (w503:T11)  [unwired: 1 in]
        n601 = Bundle("Time_Out"=w495, "Window_Spark_Rate_OUT"=w482) -> (w509:T12)  [unwired: 1 in]
        n602 = Bundle("Time_Out"=w495, "Window_Median_OUT"=w494) -> (w515:T13)  [unwired: 1 in]
        n603 = Bundle("Time_Out"=w496, "Window_Avg_OUT"=w486) -> (w504:T11)  [unwired: 1 in]
        n604 = Bundle("Time_Out"=w496, "Window_Spark_Rate_OUT"=w485) -> (w510:T12)  [unwired: 1 in]
        n605 = Bundle("Time_Out"=w496, "Window_Median_OUT"=w497) -> (w516:T13)  [unwired: 1 in]
        n606 = Bundle("Time_Out"=w498, "Window_Avg_OUT"=w488) -> (w505:T11)  [unwired: 1 in]
        n607 = Bundle("Time_Out"=w498, "Window_Spark_Rate_OUT"=w487) -> (w511:T12)  [unwired: 1 in]
        n608 = Bundle("Time_Out"=w498, "Window_Median_OUT"=w499) -> (w517:T13)  [unwired: 1 in]
        n609 = Bundle("Time_Out"=w500, "Window_Avg_OUT"=w478) -> (w506:T11)  [unwired: 1 in]
        n610 = Bundle("Time_Out"=w500, "Window_Spark_Rate_OUT"=w489) -> (w512:T12)  [unwired: 1 in]
        n611 = Bundle("Time_Out"=w500, "Window_Median_OUT"=w501) -> (w518:T13)  [unwired: 1 in]
        n612 = Build Array(w645, w644, w643, w642, w641, w640) -> (w456:T3)
        n613 = Build Array(w639, w638, w637, w636, w635, w634) -> (→"L1-Sparks/min":T4)
        n614 = Build Array(w633, w632, w631, w630, w629, w628) -> (w457:T14)
        n615 = Build Array(w610, w611, w612, w613, w614, w615) -> (w450:T3)
        n616 = Build Array(w616, w617, w618, w619, w620, w621) -> (→"L2-Sparks/min":T4)
        n617 = Build Array(w622, w623, w624, w625, w626, w627) -> (w452:T14)
        n618 = Build Array(w532, w549, w548, w547, w546, w545) -> (w447:T3)
        n619 = Build Array(w544, w543, w542, w541, w540, w539) -> (→"L3-Sparks/min":T4)
        n620 = Build Array(w538, w537, w536, w535, w534, w533) -> (w448:T14)
        n621 = Build Array(w519, w502, w503, w504, w505, w506) -> (w442:T3)
        n622 = Build Array(w507, w508, w509, w510, w511, w512) -> (→"L4-Sparks/min":T4)
        n623 = Build Array(w513, w514, w515, w516, w517, w518) -> (w444:T14)
        n624 = Select(t=w448, s="Sow_Median_L3", f=w447) -> (s? t:f=→"L3-Average/WindowSize":T3)
        n625 = Select(t=w444, s="Sow_Median_L4", f=w442) -> (s? t:f=→"L4-Average/WindowSize":T3)
        n626 = Select(t=w457, s="Sow_Median_L1", f=w456) -> (s? t:f=→"L1-Average/WindowSize":T3)
        n627 = Select(t=w452, s="Sow_Median_L2", f=w450) -> (s? t:f=→"L2-Average/WindowSize":T3)
        n628 = case shown="True" "Sow_Median_L3" {
          frame False {
            n629 = property on="L3-Average/WindowSize" class="XYGraph (strict)"("YScale.NameLbl.Text"="Avg [uA]" ("Y Scale.Name Label.Text")) -> ()  [unwired: 2 in, 2 out]
          }
          frame True {
            n630 = property on="L3-Average/WindowSize" class="XYGraph (strict)"("YScale.NameLbl.Text"="Current [uA]" ("Y Scale.Name Label.Text")) -> ()  [unwired: 2 in, 2 out]
          }
        }
        n631 = case shown="False" "Sow_Median_L4" {
          frame False {
            n632 = property on="L4-Average/WindowSize" class="XYGraph (strict)"("YScale.NameLbl.Text"="Avg [uA]" ("Y Scale.Name Label.Text")) -> ()  [unwired: 2 in, 2 out]
          }
          frame True {
            n633 = property on="L4-Average/WindowSize" class="XYGraph (strict)"("YScale.NameLbl.Text"="Current [uA]" ("Y Scale.Name Label.Text")) -> ()  [unwired: 2 in, 2 out]
          }
        }
        n634 = case shown="False" "Sow_Median_L1" {
          frame False {
            n635 = property on="L1-Average/WindowSize" class="XYGraph (strict)"("YScale.NameLbl.Text"="Avg [uA]" ("Y Scale.Name Label.Text")) -> ()  [unwired: 2 in, 2 out]
          }
          frame True {
            n636 = property on="L1-Average/WindowSize" class="XYGraph (strict)"("YScale.NameLbl.Text"="Current [uA]" ("Y Scale.Name Label.Text")) -> ()  [unwired: 2 in, 2 out]
          }
        }
        n637 = case shown="False" "Sow_Median_L2" {
          frame False {
            n638 = property on="L2-Average/WindowSize" class="XYGraph (strict)"("YScale.NameLbl.Text"="Avg [uA]" ("Y Scale.Name Label.Text")) -> ()  [unwired: 2 in, 2 out]
          }
          frame True {
            n639 = property on="L2-Average/WindowSize" class="XYGraph (strict)"("YScale.NameLbl.Text"="Current [uA]" ("Y Scale.Name Label.Text")) -> ()  [unwired: 2 in, 2 out]
          }
        }
      }
      event "L1_Horizontal Slider", "L1_Vertical Slider", "L2_Horizontal Slider", "L2_Vertical Slider", "L3_Horizontal Slider", "L3_Vertical Slider", "L4_Horizontal Slider", "L4_Vertical Slider": Value Change {
        n640 = event-data() -> ()  [unwired: 1 in, 6 out]
        n641 = Unbundle("L1_Horizontal Slider") -> ("Slider"=w1394:dbl, "Slider"=w1393:dbl)
        n642 = Unbundle("L2_Horizontal Slider") -> ("Slider"=w1391:dbl, "Slider"=w1392:dbl)
        n643 = Unbundle("L3_Horizontal Slider") -> ("Slider"=w1381:dbl, "Slider"=w1382:dbl)
        n644 = Unbundle("L4_Horizontal Slider") -> ("Slider"=w1384:dbl, "Slider"=w1383:dbl)
        n645 = Unbundle("L1_Vertical Slider") -> ("Slider"=w1396:dbl, "Slider"=w1395:dbl)
        n646 = Unbundle("L2_Vertical Slider") -> ("Slider"=w1389:dbl, "Slider"=w1390:dbl)
        n647 = Unbundle("L3_Vertical Slider") -> ("Slider"=w1379:dbl, "Slider"=w1380:dbl)
        n648 = Unbundle("L4_Vertical Slider") -> ("Slider"=w1386:dbl, "Slider"=w1385:dbl)
        n649 = property on="L1-Current_Zoomed" class="XYGraph (strict)"("YScale.Maximum"=w1396, "YScale.Minimum"=w1395) -> ()  [unwired: 2 in, 2 out]
        n650 = property on="L1-Current_Zoomed" class="XYGraph (strict)"("XScale.Maximum"=w1394, "XScale.Minimum"=w1393) -> ()  [unwired: 2 in, 2 out]
        n651 = property on="L2-Current_Zoomed" class="XYGraph (strict)"("YScale.Maximum"=w1389, "YScale.Minimum"=w1390) -> ()  [unwired: 2 in, 2 out]
        n652 = property on="L2-Current_Zoomed" class="XYGraph (strict)"("XScale.Maximum"=w1391, "XScale.Minimum"=w1392) -> ()  [unwired: 2 in, 2 out]
        n653 = property on="L3-Current_Zoomed" class="XYGraph (strict)"("YScale.Maximum"=w1379, "YScale.Minimum"=w1380) -> ()  [unwired: 2 in, 2 out]
        n654 = property on="L3-Current_Zoomed" class="XYGraph (strict)"("XScale.Maximum"=w1381, "XScale.Minimum"=w1382) -> ()  [unwired: 2 in, 2 out]
        n655 = property on="L4-Current_Zoomed" class="XYGraph (strict)"("YScale.Maximum"=w1386, "YScale.Minimum"=w1385) -> ()  [unwired: 2 in, 2 out]
        n656 = property on="L4-Current_Zoomed" class="XYGraph (strict)"("XScale.Maximum"=w1384, "XScale.Minimum"=w1383) -> ()  [unwired: 2 in, 2 out]
      }
      event "Stop": Value Change {
        n657 = event-data() -> ()  [unwired: 1 in, 6 out]
      }
      event Timeout {
        n658 = event-data() -> ()  [unwired: 1 in, 3 out]
        n659 = for {
          N: 6 -> [_]
          i -> [w1401]
          n660 = property on="L1-Current_Zoomed" class="XYGraph (strict)"("Active Plot"=w1401) -> ("Plot.Visible?"=w1405:bool)  [unwired: 2 in, 2 out]
          n661 = property on="L2-Current_Zoomed" class="XYGraph (strict)"("Active Plot"=w1401) -> ("Plot.Visible?"=w1404:bool)  [unwired: 2 in, 2 out]
          n662 = property on="L3-Current_Zoomed" class="XYGraph (strict)"("Active Plot"=w1401) -> ("Plot.Visible?"=w1403:bool)  [unwired: 2 in, 2 out]
          n663 = property on="L4-Current_Zoomed" class="XYGraph (strict)"("Active Plot"=w1401) -> ("Plot.Visible?"=w1402:bool)  [unwired: 2 in, 2 out]
          n664 = property on="L3-Current_Full" class="XYGraph (strict)"("Plot.Visible?"=w1403, "Active Plot"=w1401) -> ()  [unwired: 2 in, 2 out]
          n665 = property on="L4-Current_Full" class="XYGraph (strict)"("Plot.Visible?"=w1402, "Active Plot"=w1401) -> ()  [unwired: 2 in, 2 out]
          n666 = property on="L2-Current_Full" class="XYGraph (strict)"("Plot.Visible?"=w1404, "Active Plot"=w1401) -> ()  [unwired: 2 in, 2 out]
          n667 = property on="L1-Current_Full" class="XYGraph (strict)"("Plot.Visible?"=w1405, "Active Plot"=w1401) -> ()  [unwired: 2 in, 2 out]
        }
      }
    }
  }
